vi "GEA2_ICP_Dryer_SM.vi"(0 "ComPort":refnum<visa-resource-name>="COM1", 1 "Destination Address":u8=36 format="%.0x", 2 "Source Address":u8=229 format="%.0x", 5 "Mode":T5=enum."Simulate Dryer", 7 "Xtra Command Data":u8[](array[numeric]) format="%02x", 9 "Dryer Status Serial Data In":T3, 11 "Error In":errorcluster, 13 "Command":T2 items=["CMD_Eval_Mode_Entry_CC1", "CMD_Eval_Mode_Entry_CC2", "CMD_Eval_Mode_Continue", "CMD_Send_DIAG_Info", "CMD_Enable_Debug_Log ", "CMD_Disable_Debug_Log ", "CMD_Send_Log_Data", "CMD_Stop", "RQST_Version"]) -> (4 "Dryer Status Serial Data Out":T3={"Color"=0, "Last Read Status"=enum."Err", "Command:Data"="", "Com Port"=0, "Time(S)"=0.0, "Err Count"=0}, 6 "Read_ACK":bool, 8 "DataReturned":u8[](array[numeric]) format="%.0x", 10 "WriteOK":bool, 14 "CRC Match":bool, 15 "Error Out":errorcluster)   [LabVIEW 2009]
uses:
  GEA2 Dryer Interface Ctrl.ctl
  Dryer Commands.ctl
  Dryer Status Ctrl.ctl
  Dryer Com Port Info.ctl
  <vilib>/Instr/_visa.llb/VISA Configure Serial Port (Instr).vi
  Globals Wilt.vi
  Hybrid Water Heater/HEWH Error Enumeration.ctl
  <vilib>/regexp/Match Regular Expression.xnode
panel:
  out "Remaining States":string
  out "after substring":string
  out "return count 3":u32
  out "Current Read Index":i32
  out "return count":u32
  out "ReadCM2Flag":bool
  out "ReadCM1Flag":bool
  out "Com:Data Buffer":string
  out "Tstart":dbl format="%.2f"
  out "Com:Data":string
  out "CRCArray":u8[](array[numeric]) format="%.0x"
  in  "Tab Control":T1(tab)=enum."Simulate Dryer Data"
  in  "Sim Data":u8[](array[numeric]) format="%02x"
  out "Command Bytes":u8[](array[numeric])=[226, 96, 8, 128, 86, 123, 137, 227] format="%.0x"
  out "ACK(E1?)":u8[](array[numeric]) format="%.0x"
  out "Message Out":u8[](array[numeric]) format="%.0x"
  out "Length":u8
  out "Source Read":u8 format="%.0x"
  out "Destination Read":u8 format="%.0x"
  out "ReadArray":u8[](array[numeric]) format="%.0x"
  out "Bytes At Port":u32=40
  out "CRCRead":u8[](array[numeric]) format="%.0x"
  out "CRC Calc":u8[](array[numeric]) format="%.0x"
  out "Timeout":bool
  out "Num Messages":dbl
  out "Read Pulse":dbl
  out "Time Array":i32[](array[numeric])
  out "Tdiff":i32[](array[numeric])
  out "tStart":u32
  out "State Array":string[](array[string])
  out "Total mS":i32
  in  "Debug":bool
  out "Message for Me":bool
  out "read buffer":string
  out "Partial Message":bool
  out "Send Array":string
  in  "Dryer Status 2 Send":T4
  out "STATUS ACK":bool
  out "ASCII ACK":bool
  out "Status Count":dbl
  out "ASCII Count":dbl
  in  "Period of STATUS (Counts)":dbl=60.0
  in  "Period of Send(mS)":i32=1000
  in  "Enable Read ACK?":bool
  out "Timeout ACK":bool
  in  "Cycle Time (s)":dbl=1000.0 format="%.2f"
  out "Time Left":dbl
  in  "Sim Dryer Start":bool
  out "Drying":bool=TRUE
  out "Sim Init":bool
  out "Start Pressed":bool
  out "Wait Restart":bool
  in  "Serial Timeout":u32=10
  in  "Exit":bool
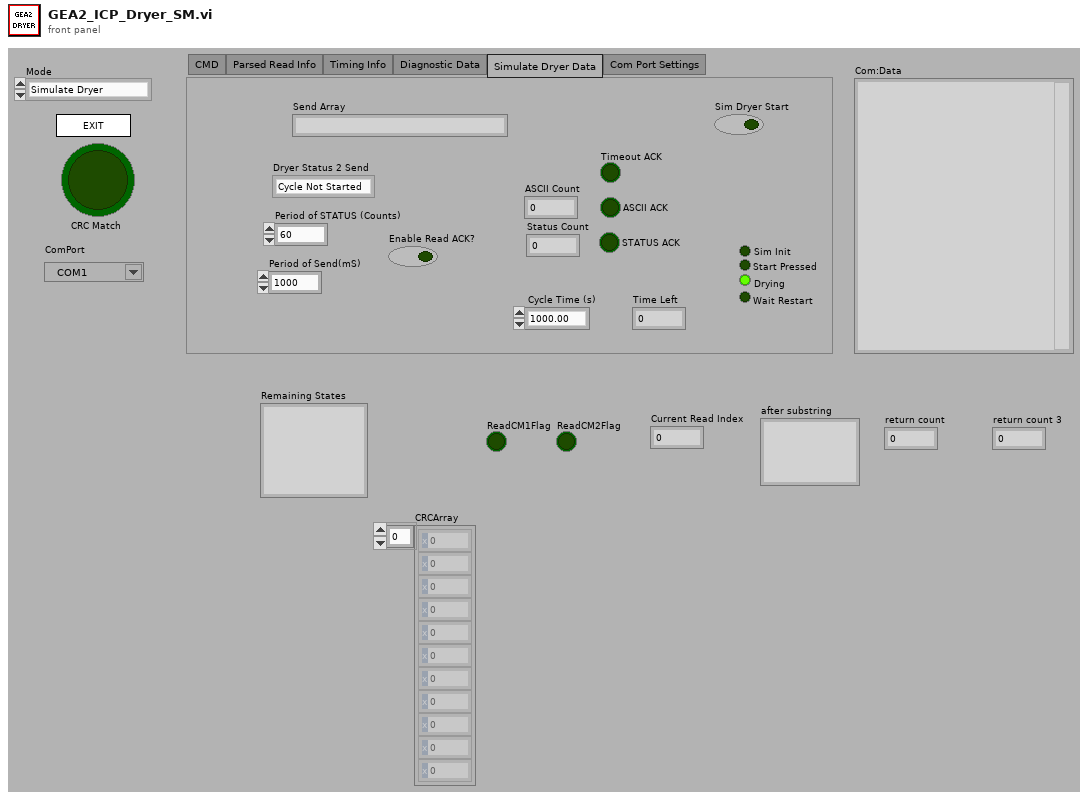
[diagram p1: front panel]
types:
  T1 = enum32{"CMD", "Parsed Read Info", "Timing Info", "Diagnostic Data", "Simulate Dryer Data", "Com Port Settings"}
  T2 = typedef "Dryer Commands.ctl" = u8
  T3 = typedef "Dryer Com Port Info.ctl" = cluster{"Color":u32, "Last Read Status":T4, "Command:Data":string, "Com Port":u8, "Time(S)":dbl, "Err Count":u32}
  T4 = typedef "Dryer Status Ctrl.ctl" = enum16{"Cycle Not Started", "Cycle Running", "Paused", "Cycle Completed", "Eval Mode Entered", "Err"}
  T5 = typedef "GEA2 Dryer Interface Ctrl.ctl" = enum16{"Init Com Port", "SendCMD", "ReadPort", "Close Port", "Simulate Diag Data", "Simulate Dryer", "Send WILT Startup CMDs", "Send Continue CMD", "Read Continuous"}
  T6 = enum32{"invalid app kind", "Development System", "Run Time System", "Student Edition", "Embedded LabVIEW", "Evaluation", "Custom"}
  T7 = enum32{"Invalid", "Standard", "Closed", "Hidden", "Minimized", "Maximized"}
  T8 = typedef "HEWH Error Enumeration.ctl" = enum16{"No Error", "GEA2 Send ACK Mismatch", "GEA2 STX", "GEA2 ETX", "GEA2 CRC Mismatch", "GEA2 ReadACK", "RTD In Range Error", "Fail Mean Tank Temp", "No Flow Config Data Found", "Failed Flow During Purge", "Temp During Purge", "Confirm IF Stop Fail", "Init Draw: TC_1 Out of Range", "Flow = 0 During Draw after 20s"}
  T9 = cluster{"Core":cluster{"Current VI Reference":refnum<vi>, "Close Panel on Exit?":bool}, "ComPort":refnum<visa-resource-name>, "ReadArray":u8[], "CRCArray":u8[], "Bytes Remaining":u8, "CRCRead":u8[], "CRC":bool, "Dryer Command":T2, "Error Out Flag":bool, "Bytes Data":u8[], "Dryer Status Serial Data In":T3, "Current Read Index":i32, "Total Bytes Read":i32, "Reset MSG Count":bool, "ACK":bool, "ReadCM1Flag":bool, "ReadCM2Flag":bool, "Reset Pulse":bool}
  T10 = cluster{"Current VI Reference":refnum<vi>, "Close Panel on Exit?":bool}
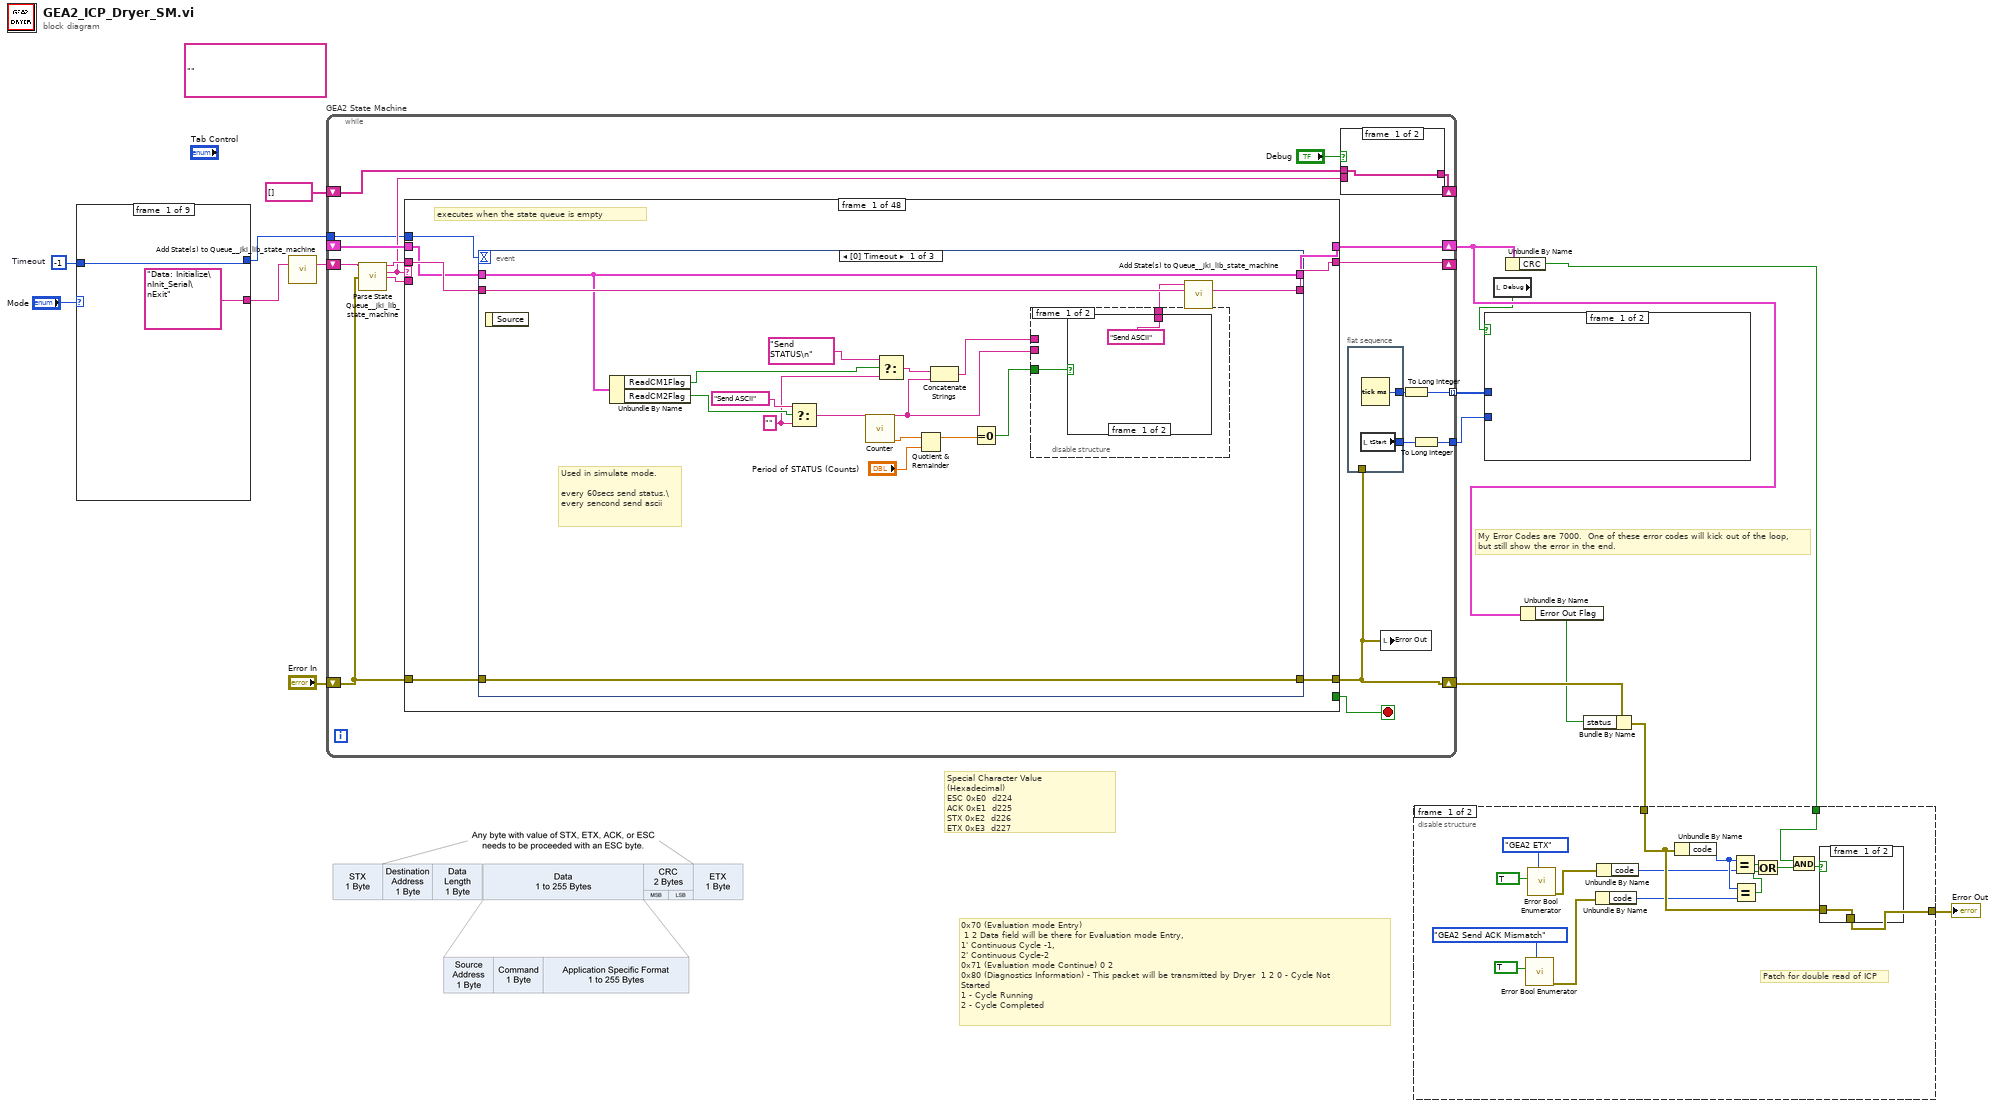
[diagram p0: block diagram]
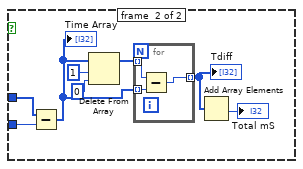
[diagram p2: hidden frame]
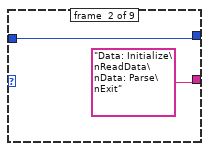
[diagram p3: hidden frame]
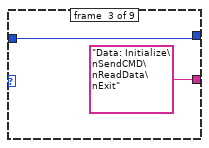
[diagram p4: hidden frame]
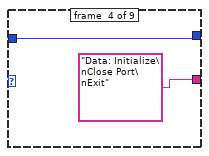
[diagram p5: hidden frame]
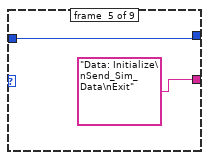
[diagram p6: hidden frame]
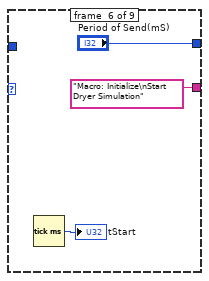
[diagram p7: hidden frame]
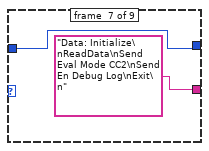
[diagram p8: hidden frame]
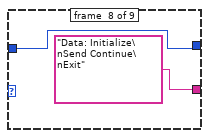
[diagram p9: hidden frame]
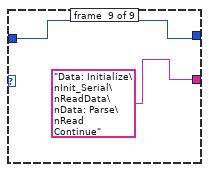
[diagram p10: hidden frame]
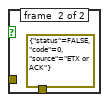
[diagram p11: hidden frame]
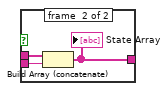
[diagram p13: hidden frame]
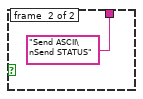
[diagram p14: hidden frame]
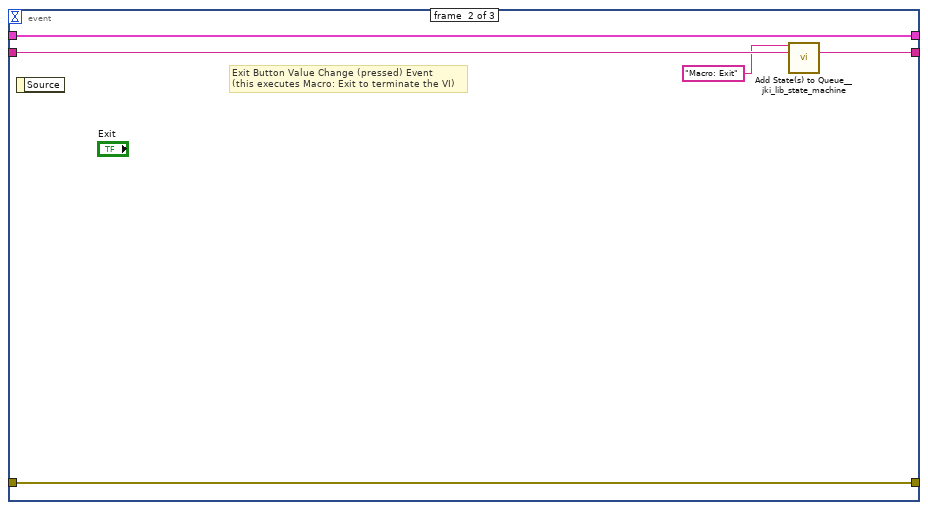
[diagram p17: hidden frame]
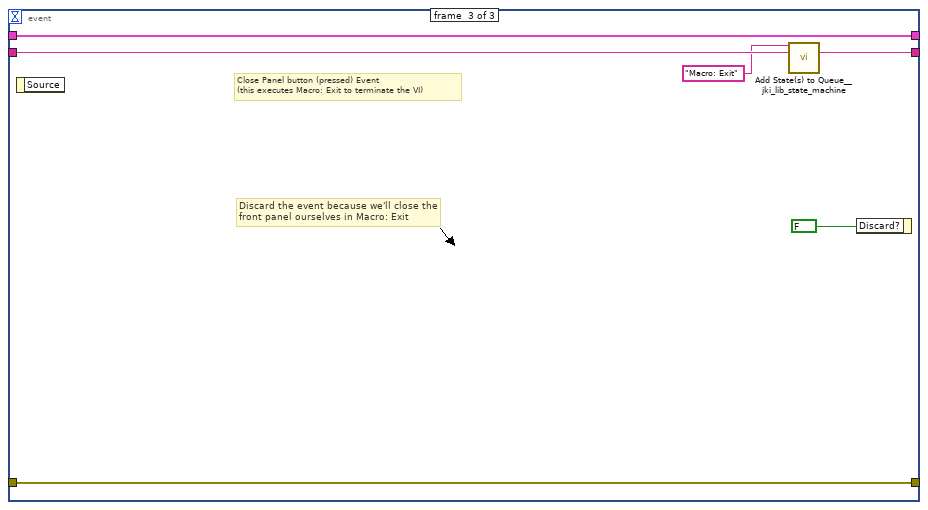
[diagram p18: hidden frame]
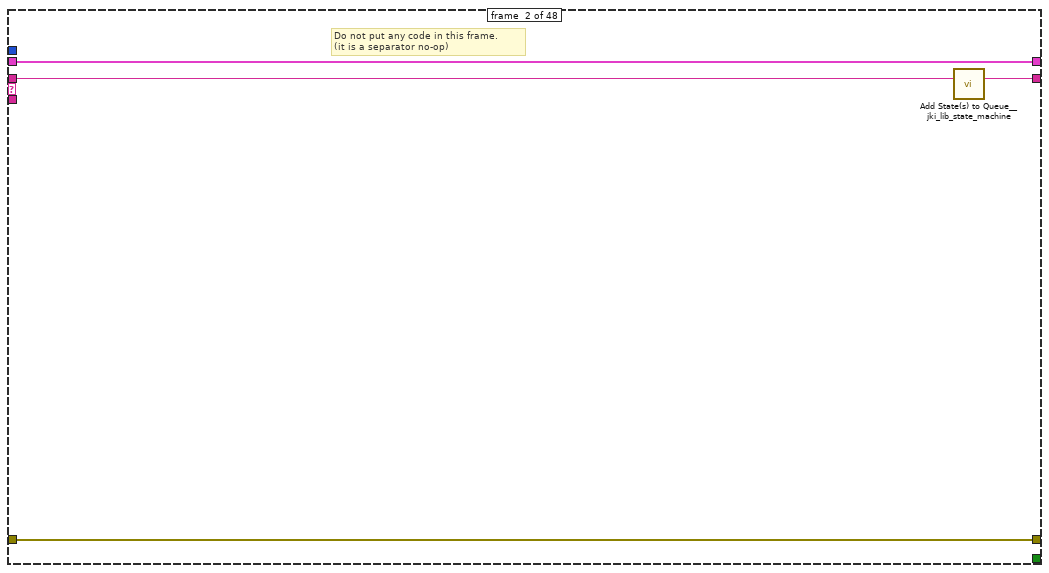
[diagram p19: hidden frame]
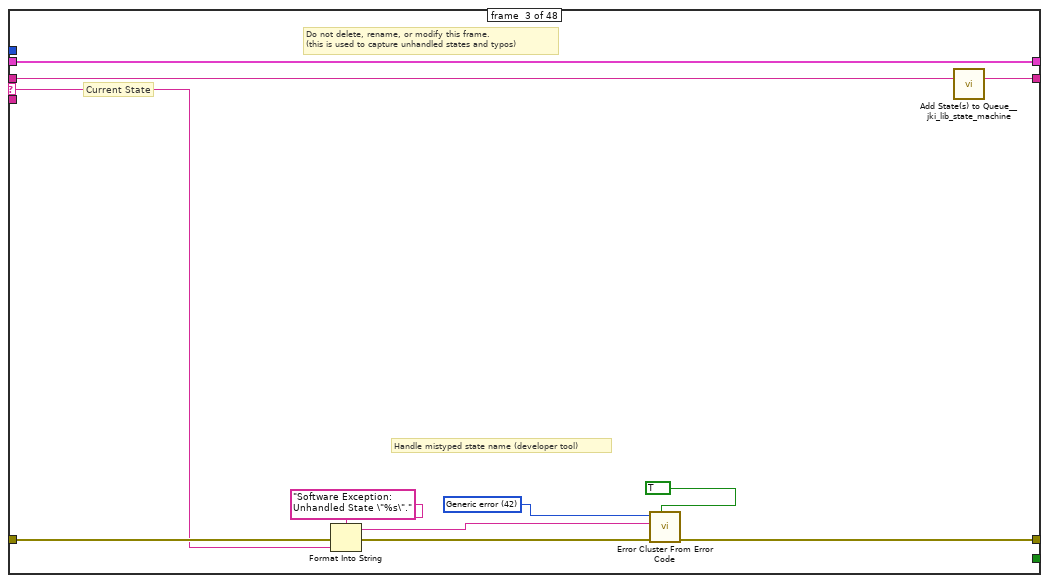
[diagram p20: hidden frame]
diagram:
  (unwired) ""
  w3 = -1  # Timeout
  # "0x70 (Evaluation mode Entry) \n\t1\t2\tData field will be there for Evaluation mode Entry, \n1' Continuous Cycle -1, \n2' Continuous Cycle-2\n0x71 (Evaluation mode Continue)\t0\t2\t\n0x80 (Diagnostics Information) - This packet will be transmitted by Dryer \t1\t2\t0 - Cycle Not Started\n1 - Cycle Running\n2 - Cycle Completed"
  # "My Error Codes are 7000.  One of these error codes will kick out of the loop,\nbut still show the error in the end."
  # "Special Character\tValue (Hexadecimal)\nESC\t0xE0  d224\nACK\t0xE1  d225\nSTX\t0xE2  d226\nETX\t0xE3  d227"
  n1 = case shown="\"ReadPort\", Default" "Mode" {
    tunnel: ["Data: Initialize\nInit_Serial\nExit" "Data: Initialize\nReadData\nData: Parse\nExit" "Data: Initialize\nSendCMD\nReadData\nExit" "Data: Initialize\nClose Port\nExit" "Data: Initialize\nSend_Sim_Data\nExit" "Macro: Initialize\nStart Dryer Simulation" "Data: Initialize\nReadData\nSend Eval Mode CC2\nSend En Debug Log\nExit\n" "Data: Initialize\nSend Continue\nExit" "Data: Initialize\nInit_Serial\nReadData\nData: Parse\nRead Continue"] -> w1
    tunnel: [w17 w19 w21 w23 w25 "Period of Send(mS)" w30 w32 w35] -> w4
    tunnel: w3 -> [w17 w19 w21 w23 w25 _ w30 w32 w35]
    frame #0 {
    }
    frame #1 {
    }
    frame #2 {
    }
    frame #3 {
    }
    frame #4 {
    }
    frame #5 {
      n2 = Tick Count (ms)() -> (millisecond timer value=→"tStart":u32)
    }
    frame #6 {
    }
    frame #7 {
    }
    frame #8 {
    }
  }
  n3 = call <vilib>:"Add State(s) to Queue__jki_lib_state_machine.vi"("State(s) in (\"\")"=w1) -> ("States Out"=w16:string)  [unwired: 14 in]
  n4 = while "GEA2 State Machine" {
    shift-right: [w49] -> w7
    shift-left: _ -> [w48]
    shift-right: [w45] -> w14
    shift-left: "Error In" -> [w47]
    shift-right: [w46] -> _
    shift-left: w16 -> [w51]
    tunnel: [w42] -> w13 mode=indexing
    tunnel: [w41] -> w12
    shift-right: [w38] -> _
    shift-left: string[] [] -> [w40]
    tunnel: w4 -> [w37]
    stop <- w50 stop-if-true
    n5 = call <vilib>:"Parse State Queue__jki_lib_state_machine.vi"("State Queue"=w51, "Error In (no error)"=w47) -> ("Remaining States"=w53:string, "Current State"=w39:string, "Arguments"=w52:string)  [unwired: 11 in]
    n6 = case shown="\"ReadData\"" w39 {
      selector: w39 -> [_ _ w109 _ _ _ _ _ _ _ _ _ _ _ _ _ _ _ _ _ _ _ _ _ _ _ _ _ _ _ _ _ _ _ _ _ _ _ _ _ _ _ _ _ _ _ _ _]
      tunnel: w53 -> [w66 w108 w113 w131 w147 w149 w164 w192 w199 w204 w208 w214 w225 w251 w256 w261 w272 w299 w324 w371 w409 w444 w481 w491 w548 w628 w663 w671 w679 w704 w740 w759 w803 w832 w853 w874 w890 w903 w916 w952 w966 w992 w1004 w1009 w1033 w1267 w1283 w1322]
      tunnel: w52 -> [_ _ _ _ _ _ _ _ _ _ _ w209 w219 _ _ _ _ _ _ _ _ _ _ _ _ _ _ _ _ _ _ _ _ _ _ _ _ _ _ _ _ _ _ _ _ _ _ _]
      tunnel: w48 -> [w64 w105 w111 w122 w143 w152 w161 _ w196 w201 w206 w212 w221 w248 w253 w258 w269 w296 w321 w343 w380 w421 w458 w486 w543 w606 w660 w668 w673 w702 w738 w775 w801 w830 w851 w872 w885 w901 w911 w946 w955 w973 w1001 w1006 w1017 w1262 w1279 w1318]
      tunnel: [w63 w106 w115 w128 w145 w153 w162 w178 w194 w202 w205 w210 w222 w249 w254 w259 w270 w297 w322 w348 w374 w412 w445 w487 w544 w611 w646 w669 w677 w699 w734 w772 w795 w826 w847 w868 w883 w898 w912 w950 w964 w990 w1002 w1007 w1031 w1265 w1282 w1320] -> w45
      tunnel: w47 -> [w62 w106 w114 w128 w139 w153 w162 w178 w197 w202 w205 w211 w223 w249 w254 w259 w270 w282 w317 w350 w393 w427 w464 w488 w545 w613 w643 w669 w677 w696 w734 w772 w795 w826 w847 w868 w888 w895 w914 w950 w964 w990 w1002 w1007 w1031 w1265 w1282 w1320]
      tunnel: [w65 w107 w112 w130 w146 w154 w163 w191 w198 w203 w207 w213 w224 w250 w255 w260 w271 w298 w323 w370 w408 w443 w480 w490 w547 w627 w662 w670 w678 w703 w739 w776 w802 w831 w852 w873 w889 w902 w915 w951 w965 w991 w1003 w1008 w1032 w1266 w1275 w1321] -> w46
      tunnel: [_ _ _ _ _ w150 _ _ _ _ _ _ _ _ _ _ _ _ _ _ _ _ _ _ _ _ _ _ _ _ _ _ _ _ _ _ _ _ _ _ _ _ _ _ _ _ _ _] -> w50
      tunnel: [w61 w105 w111 w129 w142 w152 w161 w190 w196 w201 w206 w212 w221 w248 w253 w258 w269 w295 w320 w343 w379 w421 w458 w486 w543 w606 w653 w668 w672 w701 w737 w774 w800 w829 w850 w871 w884 w900 w911 w945 w954 w989 w1001 w1006 w1014 w1262 w1279 w1318] -> w49
      tunnel: w37 -> [w60 _ _ _ _ _ _ _ _ _ _ _ _ _ _ _ _ _ _ _ _ _ _ _ _ _ _ _ _ _ _ _ _ _ _ _ _ _ _ _ _ _ _ _ _ _ _ _]
      frame #0 {
        # "executes when the state queue is empty"
        n7 = event shown="[0] Timeout" {
          selector: _ -> [_ _ _]
          dyn-events: _ -> [_ _ _]
          timeout: w60 -> [_ _ _]
          tunnel: w66 -> [w83 w98 w104]
          tunnel: [w82 w97 w103] -> w65
          tunnel: w64 -> [w75 w95 w101]
          tunnel: [w81 w96 w102] -> w63
          tunnel: w62 -> [w81 w96 w102]
          tunnel: [w75 w95 w101] -> w61
          event #0 {
            w71 = "" ("f")
            # "Used in simulate mode.\n\nevery 60secs send status.\\\nevery sencond send ascii"
            n8 = event-data() -> ()  [unwired: 1 in, 1 out]
            n9 = Unbundle By Name(w75) -> ("ReadCM1Flag"=w70:bool, "ReadCM2Flag"=w73:bool)
            n10 = Select(t="Send ASCII" ("State(s) in Front (\"\")"), s=w73, f=w71) -> (s? t:f=w68:string)
            n11 = call "Counter.vi"() -> ("Count"=w79:dbl)  [unwired: 11 in]
            n12 = Select(t="Send STATUS\n" ("State(s) in Front (\"\")"), s=w70, f=w71) -> (s? t:f=w69:string)
            n13 = Quotient & Remainder(x=w79, y="Period of STATUS (Counts)") -> (x-y*floor(x/y)=w77:dbl)  [unwired: 1 out]
            n14 = Concatenate Strings(w69, w68) -> (w67:string)
            n15 = Equal To 0?(x=w77) -> (x = 0?=w76:bool)
            n16 = disable-structure shown="Enabled" {
              disable-tunnel: [w85 w90] -> w80
              disable-tunnel: w76 -> [w84 w91]
              disable-tunnel: w68 -> [_ w89]
              disable-tunnel: w67 -> [_ w88]
              frame #0 {
                n17 = case shown="False" w84 {
                  tunnel: ["Send ASCII" ("State(s) in Front (\"\")") "Send ASCII\nSend STATUS" ("State(s) in Front (\"\")")] -> w85
                  frame #0 {
                  }
                  frame #1 {
                  }
                }
              }
              frame #1 {
                n18 = case shown="False" w91 {
                  tunnel: [w92 w93] -> w90
                  tunnel: w89 -> [w92 _]
                  tunnel: w88 -> [_ w93]
                  frame #0 {
                  }
                  frame #1 {
                  }
                }
              }
            }
            n19 = call <vilib>:"Add State(s) to Queue__jki_lib_state_machine.vi"("State(s) in Front (\"\")"=w80, "State(s) in (\"\")"=w83) -> ("States Out"=w82:string)  [unwired: 13 in]
          }
          event #1 {
            # "Exit Button Value Change (pressed) Event\n(this executes Macro: Exit to terminate the VI)"
            n20 = event-data() -> ()  [unwired: 1 in, 1 out]
            n21 = call <vilib>:"Add State(s) to Queue__jki_lib_state_machine.vi"("State(s) in Front (\"\")"="Macro: Exit", "State(s) in (\"\")"=w98) -> ("States Out"=w97:string)  [unwired: 13 in]
          }
          event #2 {
            # "Discard the event because we'll close the front panel ourselves in Macro: Exit"
            # "Close Panel button (pressed) Event\n(this executes Macro: Exit to terminate the VI)"
            n22 = event-data() -> ()  [unwired: 1 in, 1 out]
            n23 = call <vilib>:"Add State(s) to Queue__jki_lib_state_machine.vi"("State(s) in Front (\"\")"="Macro: Exit", "State(s) in (\"\")"=w104) -> ("States Out"=w103:string)  [unwired: 13 in]
            n24 = event-data("Discard?"=FALSE) -> ()  [unwired: 1 in, 1 out]
          }
        }
      }
      frame #1 {
        # "Do not put any code in this frame.\n(it is a separator no-op)"
        n25 = call <vilib>:"Add State(s) to Queue__jki_lib_state_machine.vi"("State(s) in (\"\")"=w108) -> ("States Out"=w107:string)  [unwired: 14 in]
      }
      frame #2 {
        w118 = 42 items=["No error", "Argument error", "Memory is full", "Out of zone", "End of file", "File already open", "Generic file I/O error", "File not found", "File permission error", "Disk is full", "Duplicate path", "Too many files open", "System feature not enabled", "Resource file not found", "Cannot add resource", "Resource not found", "Image not found", "Image memory error", "Pen does not exist", "Config type invalid", "Config token not found", "Config parse error", "Config memory error", "Bad external code format", "Bad external code offset", "External code not present", "Null window", "Destroy window error", "Null menu", "Print aborted", "Bad print record", "Print driver error", "Windows error during printing", "Memory error during printing", "Print dialog error", "Generic print error", "Invalid device refnum", "Device not found", "Device parameter error", "Device unit error", "Cannot open device", "Device call aborted", "Generic error", "Cancelled by user", "Object ID too low", "Object ID too high", "Object not in heap", "Unknown heap", "Unknown object (invalid DefProc)", "Unknown object (DefProc not in table)", "Message out of range", "Invalid (null) method", "Unknown message", "Manager call not supported", "Bad address", "Network operation in progress", "Network operation timed out", "Connection is busy", "Network attribute not supported", "Network error", "Address in use", "System out of memory", "Connection aborted", "Connection refused", "Not connected", "Already connected", "Connection closed", "Initialization error (interapplication manager)", "Bad occurrence", "Wait on unbound occurrence handler", "Occurrence queue overflow", "Datalog type conflict", "Unused", "Unrecognized type (interapplication manager)", "Memory corrupt", "Failed to make temporary DLL", "Old CIN version", "Drag socket not found", "Failed to load drop-object", "Failed to register OLE object", "Failed to release OLE object", "Format specifier type mismatch", "Unknown format specifier", "Too few format specifiers", "Too many format specifiers", "Scan failed", "Newer CIN version", "Error converting to variant", "Runtime menu error", "Password tampered", "Variant attribute not found", "Incompatible variant data type", "Event data is not available", "Event Store is not present", "Occurrence is not found", "Event Queue is not created", "Event info is not available", "Refnum passed is NULL", "Error retrieving Class GUID", "Error retrieving CoClass GUID", "Error retrieving TypeLib GUID.", "Bad built application magic bytes.", "Specific driver is different from the specific driver associated with the Logical Name.", "There is no session opened to the class driver.", "Max Error", "MAX - Error with config objects", "MAX - Error loading configuration", "MAX - Group not supported"]
        # "Current State"
        # "Do not delete, rename, or modify this frame.\n(this is used to capture unhandled states and typos)"
        # "Handle mistyped state name (developer tool)"
        n26 = Format Into String(format string="Software Exception: Unhandled State \"%s\"." ("message"), error in=w114, w109) -> (resulting string=w117:string, error out=w116:errorcluster)  [unwired: 1 in]
        n27 = call <vilib>:"Error Cluster From Error Code.vi"("show call chain? (False)"=TRUE, "error in (no error)"=w116, "error message (\"\")"=w117, "error code (0)"=w118) -> ("error out"=w115:errorcluster)  [unwired: 5 in]
        n28 = call <vilib>:"Add State(s) to Queue__jki_lib_state_machine.vi"("State(s) in (\"\")"=w113) -> ("States Out"=w112:string)  [unwired: 14 in]
      }
      frame #3 {
        # "Do not delete, rename, or modify this frame.\n(this is used to determine panel behavior on exit)"
        # "originally closed?"
        # "exe?"
        # "If panel starts closed or is an EXE, then close it when we exit"
        n29 = property class="VI"() -> ("Front Panel.Open"=w127:bool)  [unwired: 2 in, 2 out]
        n30 = control-ref of="Current VI Reference"() -> (w120:refnum<vi>)
        n31 = property class="App"() -> ("App.Kind"=w126:T6)  [unwired: 2 in, 2 out]
        n32 = Not(x=w127) -> (.not. x?=w124:bool)
        n33 = Equal?(x=w126, y=T6."Run Time System" ("Application:Kind")) -> (x = y?=w123:bool)
        n34 = Or(x=w124, y=w123) -> (x .or. y?=w121:bool)
        n35 = Bundle By Name(cluster=w122, "Core.Current VI Reference"=w120, "Core.Close Panel on Exit?"=w121) -> (w129:T9)
        n36 = call <vilib>:"Add State(s) to Queue__jki_lib_state_machine.vi"("State(s) in (\"\")"=w131) -> ("States Out"=w130:string)  [unwired: 14 in]
      }
      frame #4 {
        # "State Machine Does not handle having an error status = true."
        n37 = local read "ReadArray"() -> (w136:u8[])
        n38 = Unbundle By Name(w139) -> ("source"=w138:string)
        n39 = Number To Hexadecimal String(2:w136) -> (0:w135:string[])  [unwired: 1 in]
        n40 = Array To Spreadsheet String(array=w135, 3:"" ("format string")) -> (spreadsheet string=w133:string)  [unwired: 1 in]
        n41 = Concatenate Strings(w138, ":: BYTES :: " ("string"), w133) -> (w132:string)
        n42 = Bundle By Name(cluster=w143, "Error Out Flag"=TRUE) -> (w142:T9)
        n43 = Bundle By Name(cluster=w139, "source"=w132, "status"=FALSE) -> (w145:errorcluster)
        n44 = call <vilib>:"Add State(s) to Queue__jki_lib_state_machine.vi"("State(s) in Front (\"\")"="Exit", "State(s) in (\"\")"=w147) -> ("States Out"=w146:string)  [unwired: 13 in]
      }
      frame #5 {
        # "Do not put any code in this frame.\n(No errors that occur here will be handled.)"
        n45 = local read "Mode"() -> (w151:T5)
        n46 = case shown="\"Simulate Dryer\"" w151 {
          tunnel: [TRUE w160] -> w150
          tunnel: w149 -> [w155 w159]
          tunnel: [w155 w157] -> w148
          frame #0 {
          }
          frame #1 {
            (unwired) "SendACK" ("regular expression")
            n47 = Match Pattern(string=w159, regular expression="Check Complete") -> (after substring=w157:string)  [unwired: 1 in, 3 out]
            "after substring" <- w157
            n48 = local read "Exit"() -> (w160:bool)
            "Remaining States" <- w159
          }
        }
        n49 = call <vilib>:"Add State(s) to Queue__jki_lib_state_machine.vi"("State(s) in (\"\")"=w148) -> ("States Out"=w154:string)  [unwired: 14 in]
      }
      frame #6 {
        # "Do not put any code in this frame.\n(It is a separator no-op. You can make a copy of this frame to create a new Data frame)"
        n50 = call <vilib>:"Add State(s) to Queue__jki_lib_state_machine.vi"("State(s) in (\"\")"=w164) -> ("States Out"=w163:string)  [unwired: 14 in]
      }
      frame #7 {
        w165 = FALSE ("Start Pressed")
        w166 = TRUE  # Reset Pulse
        w169 = FALSE  # ReadCM2Flag
        w170 = FALSE  # ReadCM1Flag
        w167 = "" ("Com:Data")
        w171 = FALSE  # ACK
        w172 = TRUE  # Reset MSG Count
        w173 = 0  # Total Bytes Read
        w174 = 0  # Current Read Index
        w179 = u8 0 ("Length")
        w180 = T2 3 items=["Eval_Mode_Entry_CC1", "Eval_Mode_Entry_CC2", "Eval_Mode_Continue", "Get_Diagnostic_Info"]  # Dryer Command
        w181 = u8[] []  # Bytes Data
        w182 = T10 {"Current VI Reference"=refnum, "Close Panel on Exit?"=FALSE}  # Core
        w168 = FALSE ("CRC Match")
        w183 = FALSE  # Error Out Flag
        w184 = FALSE  # CRC
        w185 = u8[] []  # CRCRead
        w186 = u8 0  # Bytes Remaining
        w187 = u8[] []  # CRCArray
        w188 = u8[] []  # ReadArray
        # "Don' Run with Err In"
        # "Initialize the shift-register data, here.\n(data names are defined by what you wire into the bundle function)"
        n51 = local write "Com:Data Buffer"(w167) -> ()
        n52 = local write "Num Messages"(0.0 ("Num Messages")) -> ()
        n53 = local write "Com:Data"(w167) -> ()
        n54 = local write "Wait Restart"(w165) -> ()
        n55 = local write "Sim Init"(w165) -> ()
        n56 = local write "Start Pressed"(w165) -> ()
        n57 = local write "Drying"(w165) -> ()
        n58 = local write "ReadCM2Flag"(w165) -> ()
        n59 = local write "Exit"(w165) -> ()
        n60 = local write "ReadCM1Flag"(w165) -> ()
        n61 = local write "Source Read"(w179) -> ()
        n62 = local write "Length"(w179) -> ()
        n63 = local write "Message for Me"(w168) -> ()
        n64 = local write "Message for Me"(w168) -> ()
        n65 = local write "CRC Match"(w168) -> ()
        n66 = local write "WriteOK"(w168) -> ()
        n67 = local write "Read_ACK"(w168) -> ()
        n68 = local write "Timeout"(w168) -> ()
        n69 = local write "Partial Message"(w168) -> ()
        n70 = local write "Drying"(w168) -> ()
        n71 = Bundle("Core"=w182, "ComPort"="ComPort", "ReadArray"=w188, "CRCArray"=w187, "Bytes Remaining"=w186, "CRCRead"=w185, "CRC"=w184, "Dryer Command"=w180, "Error Out Flag"=w183, "Bytes Data"=w181, "Dryer Status Serial Data In"="Dryer Status Serial Data In", "Current Read Index"=w174, "Total Bytes Read"=w173, "Reset MSG Count"=w172, "ACK"=w171, "ReadCM1Flag"=w170, "ReadCM2Flag"=w169, "Reset Pulse"=w166) -> (w190:T9)  [unwired: 1 in]
        n72 = case shown="Error" w178 {
          tunnel: [_ "Exit"] -> w177
          frame #0 {
          }
          frame #1 {
          }
        }
        n73 = call <vilib>:"Add State(s) to Queue__jki_lib_state_machine.vi"("State(s) in Front (\"\")"=w177, "State(s) in (\"\")"=w192) -> ("States Out"=w191:string)  [unwired: 13 in]
        "Com:Data Buffer" <- w167
      }
      frame #8 {
        # "Cleanup any data and references, here.\n(this is called automatically, by the Macro: Exit)"
        n74 = Unbundle By Name(w196) -> ("Core.Current VI Reference"=w195:refnum<vi>)
        n75 = Close Reference(reference=w195, error in (no error)=w197) -> (error out=w194:errorcluster)
        n76 = case shown="Error" w194 {
          frame #0 {
          }
          frame #1 {
            n77 = String Length(string="") -> ()  [unwired: 1 out]
          }
        }
        n78 = call <vilib>:"Add State(s) to Queue__jki_lib_state_machine.vi"("State(s) in (\"\")"=w199) -> ("States Out"=w198:string)  [unwired: 14 in]
      }
      frame #9 {
        # "Do not put any code in this frame.\n(It is a separator no-op. You can make a copy of this frame to create a new UI frame)"
        n79 = call <vilib>:"Add State(s) to Queue__jki_lib_state_machine.vi"("State(s) in (\"\")"=w204) -> ("States Out"=w203:string)  [unwired: 14 in]
      }
      frame #10 {
        # "Initialize the User Interface, here.\n(this is called automatically, by the Macro: Init)"
        n80 = call <vilib>:"Add State(s) to Queue__jki_lib_state_machine.vi"("State(s) in (\"\")"=w208) -> ("States Out"=w207:string)  [unwired: 14 in]
      }
      frame #11 {
        # "Argument"
        # "Set and Unset Cursor Busy.\n(Usage: \"UI: Cursor Set >> Busy|Idle\")"
        n81 = case shown="\"Idle\", Default" w209 {
          tunnel: w211 -> [w216 w218]
          tunnel: [w215 w217] -> w210
          frame #0 {
            n82 = call <vilib>:"Unset Busy.vi"("error in (no error)"=w216) -> ("error out"=w215:errorcluster)  [unwired: 10 in]
          }
          frame #1 {
            n83 = call <vilib>:"Set Busy.vi"("error in (no error)"=w218) -> ("error out"=w217:errorcluster)  [unwired: 9 in, 1 out]
          }
        }
        n84 = call <vilib>:"Add State(s) to Queue__jki_lib_state_machine.vi"("State(s) in (\"\")"=w214) -> ("States Out"=w213:string)  [unwired: 14 in]
      }
      frame #12 {
        # "Argument"
        # "Set Front Panel Open or Closed\n(Usage: \"UI: Front Panel State >> Open|Close\")"
        n85 = Unbundle By Name(w221) -> ("Core.Current VI Reference"=w220:refnum<vi>)
        n86 = case shown="\"Close\"" w219 {
          tunnel: w223 -> [w229 w242]
          tunnel: [w231 w243] -> w222
          tunnel: w220 -> [w230 w240]
          frame #0 {
            n87 = property class="VI"(reference=w230, error in=w229) -> (reference out=w227:refnum<vi>, error out=w228:errorcluster, "Front Panel.Open"=w226:bool)
            n88 = case shown="False" w226 {
              tunnel: [w234 w237] -> w231
              tunnel: w228 -> [w233 w237]
              tunnel: w227 -> [w232 _]
              frame #0 {
                n89 = invoke class="VI" method="FP.Open"(reference=w232, error in=w233, "Activate"=TRUE, "State"=T7."Standard") -> (error out=w234:errorcluster)  [unwired: 1 in, 4 out]
              }
              frame #1 {
              }
            }
          }
          frame #1 {
            n90 = property class="VI"(reference=w240, error in=w242) -> (reference out=w239:refnum<vi>, error out=w241:errorcluster, "Front Panel.Open"=w238:bool)
            n91 = case shown="True" w238 {
              tunnel: [w244 w247] -> w243
              tunnel: w241 -> [w244 w246]
              tunnel: w239 -> [_ w245]
              frame #0 {
              }
              frame #1 {
                n92 = invoke class="VI" method="FP.Close"(reference=w245, error in=w246) -> (error out=w247:errorcluster)  [unwired: 1 in, 2 out]
              }
            }
          }
        }
        n93 = call <vilib>:"Add State(s) to Queue__jki_lib_state_machine.vi"("State(s) in (\"\")"=w225) -> ("States Out"=w224:string)  [unwired: 14 in]
      }
      frame #13 {
        # "Do not put any code in this frame.\n(It is a separator no-op. You can make a copy of this frame to create a new Macro frame)"
        n94 = call <vilib>:"Add State(s) to Queue__jki_lib_state_machine.vi"("State(s) in (\"\")"=w251) -> ("States Out"=w250:string)  [unwired: 14 in]
      }
      frame #14 {
        w252 = "Data: Initialize\nInitialize Core Data\nUI: Initialize\nUI: Front Panel State >> Open\nInit_Serial"  # Data: Initialize Initialize Core Data UI: Initialize UI: Front Panel State >> Open Init_Serial
        # "Initialization Macro\n(This is called once, when the VI starts)"
        n95 = call <vilib>:"Add State(s) to Queue__jki_lib_state_machine.vi"("State(s) in Front (\"\")"=w252, "State(s) in (\"\")"=w256) -> ("States Out"=w255:string)  [unwired: 13 in]
      }
      frame #15 {
        # "Exit Macro\n(This is called once, when the VI exits)"
        n96 = disable-structure shown="Enabled" {
          disable-tunnel: w258 -> [w268 _]
          disable-tunnel: [w263 _] -> w257
          frame #0 {
            n97 = Unbundle By Name(w268) -> ()  [unwired: 1 out]
            n98 = Select(t="UI: Front Panel State >> Close", s=FALSE, f="") -> (s? t:f=w265:string)
            n99 = call <vilib>:"Add State(s) to Queue__jki_lib_state_machine.vi"("State(s) in (\"\")"=w265, "State(s) at Back (\"\")"="Data: Cleanup\nExit") -> ("States Out"=w263:string)  [unwired: 13 in]
          }
          frame #1 {
          }
        }
        n100 = call <vilib>:"Add State(s) to Queue__jki_lib_state_machine.vi"("State(s) in Front (\"\")"=w257, "State(s) in (\"\")"=w261) -> ("States Out"=w260:string)  [unwired: 13 in]
      }
      frame #16 {
        # "Template Separator\n(You can make a copy of, or modify, this frame)"
        n101 = call <vilib>:"Add State(s) to Queue__jki_lib_state_machine.vi"("State(s) in (\"\")"=w272) -> ("States Out"=w271:string)  [unwired: 14 in]
      }
      frame #17 {
        w289 = u16 0 items=["None", "XON/XOFF", "RTS/CTS", "XON/XOFF & RTS/CTS", "DTR/DSR", "XON/XOFF & DTR/DSR"] ("flow control (0:none)")
        w288 = u16 10 items=["1.0"=10, "1.5"=15, "2.0"=20] ("stop bits (10: 1 bit)")
        # "skip error handle routine"
        # "Assumes that if the serial port is 19200, then it is all ok."
        # "Your code here.\n(You can make a copy of, or modify, this frame)"
        n102 = Unbundle By Name(w296) -> ("ComPort"=w276:refnum<visa-resource-name>)
        n103 = call "Com Chan Type Conversion.vi"("Com Chan In"=w276) -> ("Com Channel #"=w275:u8)  [unwired: 11 in, 3 out]
        n104 = global read "Globals Wilt.vi" "No Com Color"() -> (w281:u32)
        n105 = Bundle By Name(cluster=T3 {"Color"=0, "Last Read Status"=enum."Err", "Command:Data"="", "Com Port"=0, "Time(S)"=0.0, "Err Count"=0} ("Dryer Status Serial Data Out"), "Color"=w281, "Last Read Status"=Dryer_Status_Ctrl."Err", "Command:Data"="", "Com Port"=w275, "Time(S)"=0.0, "Err Count"=u32 0) -> (w274:T3)
        n106 = call-poly "VISA Configure Serial Port"("VISA resource name"=w276, "timeout (10sec)"="Serial Timeout", "Enable Termination\nChar (T)"=FALSE ("Enable Termination\nChar (T)"), "baud rate (9600)"=u32 19200, "data bits (8)"=u16 8, "parity (0:none)"=enum16{"None", "Odd", "Even", "Mark", "Space"}."None", "error in (no error)"=w282, "stop bits (10: 1 bit)"=w288, "flow control (0:none)"=w289) -> ("VISA resource name out"=w292:refnum<visa-resource-name>, "error out"=w293:errorcluster)  [unwired: 5 in]
        n107 = Equal To 0?(x="Serial Timeout") -> (x = 0?=w284:bool)
        n108 = case shown="True" w284 {
          tunnel: w293 -> [w300 w303]
          tunnel: w292 -> [_ w302]
          tunnel: [w300 w301] -> w291
          frame #0 {
          }
          frame #1 {
            n109 = VISA Flush I/O Buffer(VISA resource name=w302, error in (no error)=w303) -> (error out=w301:errorcluster)  [unwired: 1 in, 1 out]
          }
        }
        n110 = local write "Dryer Status Serial Data Out"(w274) -> ()
        n111 = case shown="Error" w291 {
          selector: w291 -> [w304 w311]
          tunnel: w296 -> [w308 w315]
          tunnel: [w307 w314] -> w295
          tunnel: w292 -> [w306 _]
          tunnel: ["" ("State(s) in Front (\"\")") "Exit" ("State(s) in Front (\"\")")] -> w294
          tunnel: [w304 w309] -> w297
          frame #0 {
            n112 = Bundle By Name(cluster=w308, "ComPort"=w306) -> (w307:T9)
          }
          frame #1 {
            n113 = Bundle By Name(cluster=w315, "Error Out Flag"=TRUE) -> (w314:T9)
            n114 = Bundle By Name(cluster=w311, "status"=FALSE) -> (w309:errorcluster)
          }
        }
        n115 = call <vilib>:"Add State(s) to Queue__jki_lib_state_machine.vi"("State(s) in Front (\"\")"=w294, "State(s) in (\"\")"=w299) -> ("States Out"=w298:string)  [unwired: 13 in]
      }
      frame #18 {
        # "skip error handle routine"
        # "Assumes that if the serial port is 19200, then it is all ok."
        # "Your code here.\n(You can make a copy of, or modify, this frame)"
        n116 = Unbundle By Name(w321) -> ("ComPort"=w316:refnum<visa-resource-name>)
        n117 = VISA Close(VISA resource name=w316, error in (no error)=w317) -> (error out=w318:errorcluster)
        n118 = case shown="Error" w318 {
          selector: w318 -> [w326 w330]
          tunnel: w321 -> [w325 w334]
          tunnel: [w325 w333] -> w320
          tunnel: ["" ("State(s) in Front (\"\")") "Macro: Exit" ("State(s) in Front (\"\")")] -> w319
          tunnel: [w326 w328] -> w322
          frame #0 {
          }
          frame #1 {
            n119 = Bundle By Name(cluster=w334, "Error Out Flag"=TRUE) -> (w333:T9)
            n120 = Bundle By Name(cluster=w330, "status"=FALSE) -> (w328:errorcluster)
          }
        }
        n121 = call <vilib>:"Add State(s) to Queue__jki_lib_state_machine.vi"("State(s) in Front (\"\")"=w319, "State(s) in (\"\")"=w324) -> ("States Out"=w323:string)  [unwired: 13 in]
      }
      frame #19 {
        w345 = u8 225  # ACK
        w356 = u8 227  # ETX
        w359 = u8 226  # STX
        n122 = Unbundle By Name(w343) -> ("ComPort"=w369:refnum<visa-resource-name>)
        n123 = call "Dryer_DSM_CMD.vi"("Command"="Command") -> ("CMD Array"=w361:u8[])  [unwired: 10 in]
        n124 = Array Size(array=w361) -> (size(s)=w367:i32)
        n125 = Array Size(array="Xtra Command Data") -> (size(s)=w365:i32)
        n126 = Compound Arithmetic op=ADD(7 ("x"), w367, w365) -> (w363:i32)
        n127 = To Unsigned Byte Integer(number=w363) -> (unsigned 8bit integer=w364:u8)
        n128 = Build Array (concatenate)("Destination Address", w364, "Source Address", w361, "Xtra Command Data") -> (w358:u8[])
        n129 = call "crc16-ccitt (x1021).vi"("unsigned byte array"=w358) -> ("CRC"=w357:u8[])  [unwired: 9 in, 1 out]
        n130 = call "HEWH Command Needs Read.vi"("Command"="Command") -> ("RQST"=w341:bool)  [unwired: 13 in, 1 out]
        n131 = Build Array (concatenate)(w359, w358, w357, w356) -> (w338:u8[])
        n132 = call "GEA2 Add ESC Char.vi"("Message"=w338) -> ("Message Out"=w337:u8[])  [unwired: 14 in]
        "Command Bytes" <- w337
        n133 = Byte Array To String(unsigned byte array=w337) -> (string=w339:string)
        n134 = Array Size(array=w337) -> (size(s)=w352:i32)
        n135 = Increment(x=w352) -> (x+1=w346:i32)
        n136 = VISA Write(VISA resource name=w369, write buffer=w339, error in (no error)=w350) -> (VISA resource name out=w355:refnum<visa-resource-name>, error out=w354:errorcluster)  [unwired: 1 out]
        n137 = To Unsigned Long Integer(number=w346) -> (unsigned 32bit integer=w336:u32)
        n138 = Build Array (concatenate)(w337, w345) -> (w344:u8[])
        n139 = Byte Array To String(unsigned byte array=w344) -> (string=w351:string)
        n140 = VISA Read(VISA resource name=w355, byte count=w336, error in (no error)=w354) -> (read buffer=w335:string, error out=w349:errorcluster)  [unwired: 2 out]
        n141 = Equal?(x=w351, y=w335) -> (x = y?=→"WriteOK":bool)
        n142 = case shown="True" w341 {
          tunnel: ["" "ReadData\nData: Parse\n"] -> w340
          frame #0 {
          }
          frame #1 {
          }
        }
        n143 = call "Delay mS.vi"("Error In"=w349, "milliseconds to wait"=u32 10) -> ("Error Out"=w348:errorcluster)  [unwired: 13 in]
        n144 = call <vilib>:"Add State(s) to Queue__jki_lib_state_machine.vi"("State(s) in Front (\"\")"=w340, "State(s) in (\"\")"=w371) -> ("States Out"=w370:string)  [unwired: 13 in]
      }
      frame #20 {
        w389 = T2 1 items=["CMD_Eval_Mode_Entry_CC1", "CMD_Eval_Mode_Entry_CC2", "CMD_Eval_Mode_Continue", "CMD_Send_DIAG_Info", "CMD_Enable_Debug_Log ", "CMD_Disable_Debug_Log ", "CMD_Send_Log_Data"] ("Command 2")
        w391 = u8 225  # ACK
        w398 = u8 227  # ETX
        w401 = u8 226  # STX
        n145 = Unbundle By Name(w380) -> ("ComPort"=w407:refnum<visa-resource-name>)
        n146 = call "Dryer_DSM_CMD.vi"("Command"=w389) -> ("CMD Array"=w402:u8[])  [unwired: 10 in]
        n147 = local read "Destination Address"() -> (w388:u8)
        n148 = local read "Source Address"() -> (w387:u8)
        n149 = Array Size(array=w402) -> (size(s)=w406:i32)
        n150 = Compound Arithmetic op=ADD(7 ("x"), w406) -> (w403:i32)
        n151 = To Unsigned Byte Integer(number=w403) -> (unsigned 8bit integer=w404:u8)
        n152 = Build Array (concatenate)(w388, w404, w387, w402) -> (w400:u8[])
        n153 = call "crc16-ccitt (x1021).vi"("unsigned byte array"=w400) -> ("CRC"=w399:u8[])  [unwired: 9 in, 1 out]
        n154 = Build Array (concatenate)(w401, w400, w399, w398) -> (w384:u8[])
        n155 = call "GEA2 Add ESC Char.vi"("Message"=w384) -> ("Message Out"=w383:u8[])  [unwired: 14 in]
        "Message Out" <- w383
        n156 = Array Size(array=w383) -> (size(s)=w395:i32)
        n157 = Byte Array To String(unsigned byte array=w383) -> (string=w386:string)
        n158 = VISA Write(VISA resource name=w407, write buffer=w386, error in (no error)=w393) -> (VISA resource name out=w397:refnum<visa-resource-name>, error out=w396:errorcluster)  [unwired: 1 out]
        n159 = Increment(x=w395) -> (x+1=w392:i32)
        n160 = call "Delay mS.vi"("Error In"=w396, "milliseconds to wait"=u32 1000) -> ("Error Out"=w376:errorcluster)  [unwired: 13 in]
        n161 = To Unsigned Long Integer(number=w392) -> (unsigned 32bit integer=w385:u32)
        n162 = Build Array (concatenate)(w383, w391) -> (w390:u8[])
        n163 = Byte Array To String(unsigned byte array=w390) -> (string=w394:string)
        n164 = VISA Read(VISA resource name=w397, byte count=w385, error in (no error)=w376) -> (read buffer=w381:string, return count=→"return count 3":u32, error out=w382:errorcluster)  [unwired: 1 out]
        n165 = Equal?(x=w394, y=w381) -> (x = y?=w378:bool)
        n166 = Bundle By Name(cluster=w380, "ACK"=w378) -> (w379:T9)
        n167 = disable-structure shown="Enabled" {
          disable-tunnel: w382 -> [w411 _]
          disable-tunnel: [w410 _] -> w374
          frame #0 {
            n168 = call <vilib>:"Clear Errors.vi"("error in (no error)"=w411) -> ("error out"=w410:errorcluster)  [unwired: 6 in]
          }
          frame #1 {
          }
        }
        n169 = call <vilib>:"Add State(s) to Queue__jki_lib_state_machine.vi"("State(s) in (\"\")"=w409) -> ("States Out"=w408:string)  [unwired: 14 in]
      }
      frame #21 {
        w420 = T2 2 items=["CMD_Eval_Mode_Entry_CC1", "CMD_Eval_Mode_Entry_CC2", "CMD_Eval_Mode_Continue", "CMD_Send_DIAG_Info", "CMD_Enable_Debug_Log ", "CMD_Disable_Debug_Log ", "CMD_Send_Log_Data"] ("Command 2")
        w423 = u8 225  # ACK
        w433 = u8 227  # ETX
        w436 = u8 226  # STX
        n170 = Unbundle By Name(w421) -> ("ComPort"=w442:refnum<visa-resource-name>)
        n171 = call "Dryer_DSM_CMD.vi"("Command"=w420) -> ("CMD Array"=w437:u8[])  [unwired: 10 in]
        n172 = local read "Source Address"() -> (w418:u8)
        n173 = Array Size(array=w437) -> (size(s)=w441:i32)
        n174 = local read "Destination Address"() -> (w419:u8)
        n175 = Compound Arithmetic op=ADD(7 ("x"), w441) -> (w438:i32)
        n176 = To Unsigned Byte Integer(number=w438) -> (unsigned 8bit integer=w439:u8)
        n177 = Build Array (concatenate)(w419, w439, w418, w437) -> (w435:u8[])
        n178 = call "crc16-ccitt (x1021).vi"("unsigned byte array"=w435) -> ("CRC"=w434:u8[])  [unwired: 9 in, 1 out]
        n179 = Build Array (concatenate)(w436, w435, w434, w433) -> (w416:u8[])
        n180 = call "GEA2 Add ESC Char.vi"("Message"=w416) -> ("Message Out"=w414:u8[])  [unwired: 14 in]
        n181 = Array Size(array=w414) -> (size(s)=w429:i32)
        n182 = Byte Array To String(unsigned byte array=w414) -> (string=w415:string)
        n183 = Increment(x=w429) -> (x+1=w424:i32)
        n184 = VISA Write(VISA resource name=w442, write buffer=w415, error in (no error)=w427) -> (VISA resource name out=w432:refnum<visa-resource-name>, error out=w430:errorcluster)  [unwired: 1 out]
        n185 = To Unsigned Long Integer(number=w424) -> (unsigned 32bit integer=w413:u32)
        n186 = Build Array (concatenate)(w414, w423) -> (w422:u8[])
        n187 = Byte Array To String(unsigned byte array=w422) -> (string=w428:string)
        n188 = VISA Read(VISA resource name=w432, byte count=w413, error in (no error)=w430) -> (read buffer=w431:string, error out=w426:errorcluster)  [unwired: 2 out]
        n189 = Equal?(x=w428, y=w431) -> (x = y?=w417:bool)
        n190 = call "Delay mS.vi"("Error In"=w426, "milliseconds to wait"=u32 100) -> ("Error Out"=w412:errorcluster)  [unwired: 13 in]
        n191 = local write "WriteOK"(w417) -> ()
        n192 = call <vilib>:"Add State(s) to Queue__jki_lib_state_machine.vi"("State(s) in (\"\")"=w444) -> ("States Out"=w443:string)  [unwired: 14 in]
      }
      frame #22 {
        w457 = T2 4 items=["CMD_Eval_Mode_Entry_CC1", "CMD_Eval_Mode_Entry_CC2", "CMD_Eval_Mode_Continue", "CMD_Send_DIAG_Info", "CMD_Enable_Debug_Log ", "CMD_Disable_Debug_Log ", "CMD_Send_Log_Data"] ("Command 2")
        w460 = u8 225  # ACK
        w470 = u8 227  # ETX
        w473 = u8 226  # STX
        n193 = Unbundle By Name(w458) -> ("ComPort"=w479:refnum<visa-resource-name>, "ACK"=w448:bool)
        n194 = call "Dryer_DSM_CMD.vi"("Command"=w457) -> ("CMD Array"=w474:u8[])  [unwired: 10 in]
        n195 = Array Size(array=w474) -> (size(s)=w478:i32)
        n196 = local read "Destination Address"() -> (w456:u8)
        n197 = local read "Source Address"() -> (w455:u8)
        n198 = Compound Arithmetic op=ADD(7 ("x"), w478) -> (w475:i32)
        n199 = To Unsigned Byte Integer(number=w475) -> (unsigned 8bit integer=w476:u8)
        n200 = Build Array (concatenate)(w456, w476, w455, w474) -> (w472:u8[])
        n201 = call "crc16-ccitt (x1021).vi"("unsigned byte array"=w472) -> ("CRC"=w471:u8[])  [unwired: 9 in, 1 out]
        n202 = Build Array (concatenate)(w473, w472, w471, w470) -> (w452:u8[])
        n203 = call "GEA2 Add ESC Char.vi"("Message"=w452) -> ("Message Out"=w451:u8[])  [unwired: 14 in]
        n204 = Build Array (concatenate)(w451, w460) -> (w459:u8[])
        n205 = Array Size(array=w451) -> (size(s)=w466:i32)
        n206 = Increment(x=w466) -> (x+1=w461:i32)
        n207 = Byte Array To String(unsigned byte array=w459) -> (string=w465:string)
        n208 = Byte Array To String(unsigned byte array=w451) -> (string=w454:string)
        n209 = To Unsigned Long Integer(number=w461) -> (unsigned 32bit integer=w453:u32)
        n210 = VISA Write(VISA resource name=w479, write buffer=w454, error in (no error)=w464) -> (VISA resource name out=w469:refnum<visa-resource-name>, error out=w467:errorcluster)  [unwired: 1 out]
        n211 = VISA Read(VISA resource name=w469, byte count=w453, error in (no error)=w467) -> (read buffer=w468:string, return count=→"return count":u32, error out=w463:errorcluster)  [unwired: 1 out]
        n212 = Equal?(x=w465, y=w468) -> (x = y?=w450:bool)
        n213 = call "Delay mS.vi"("Error In"=w463, "milliseconds to wait"=u32 500) -> ("Error Out"=w446:errorcluster)  [unwired: 13 in]
        n214 = And(x=w448, y=w450) -> (x .and. y?=w449:bool)
        n215 = disable-structure shown="Enabled" {
          disable-tunnel: w446 -> [w483 _]
          disable-tunnel: [w482 _] -> w445
          frame #0 {
            n216 = call <vilib>:"Clear Errors.vi"("error in (no error)"=w483) -> ("error out"=w482:errorcluster)  [unwired: 6 in]
          }
          frame #1 {
          }
        }
        n217 = local write "WriteOK"(w449) -> ()
        n218 = call <vilib>:"Add State(s) to Queue__jki_lib_state_machine.vi"("State(s) in (\"\")"=w481) -> ("States Out"=w480:string)  [unwired: 14 in]
      }
      frame #23 {
        n219 = call "Counter.vi"() -> ("Count"=w484:dbl)  [unwired: 11 in]
        n220 = Unbundle By Name(w486) -> ("ComPort"=w489:refnum<visa-resource-name>)
        n221 = for {
          N: 2 -> [_]
          tunnel: w489 -> [w531]
          tunnel: w488 -> [w515]
          tunnel: [w514] -> w487
          tunnel: w484 -> [w502]
          stop <- w503 stop-if-true
          w501 = errorcluster {"status"=TRUE, "code"=-1073807339, "source"="VISA Read in GEA2_ICP_Dryer_SM.vi"}  # timeout error
          w510 = T2 6 items=["CMD_Eval_Mode_Entry_CC1", "CMD_Eval_Mode_Entry_CC2", "CMD_Eval_Mode_Continue", "CMD_Send_DIAG_Info", "CMD_Enable_Debug_Log ", "CMD_Disable_Debug_Log ", "CMD_Send_Log_Data"] ("Command")
          w512 = u8 225  # ACK
          w521 = u8 227  # ETX
          w524 = u8 226  # STX
          n222 = call "Dryer_DSM_CMD.vi"("Command"=w510) -> ("CMD Array"=w525:u8[])  [unwired: 10 in]
          n223 = local read "Destination Address"() -> (w504:u8)
          n224 = Array Size(array=w525) -> (size(s)=w530:i32)
          n225 = local read "Source Address"() -> (w505:u8)
          n226 = Quotient & Remainder(x=w502, y=32.0) -> (x-y*floor(x/y)=w506:dbl)  [unwired: 1 out]
          n227 = String To Byte Array(string="1234567890ABCDEFGHIJKLMNOPQRSTUV") -> (unsigned byte array=w508:u8[])
          n228 = Rotate 1D Array(1:w508, 2:w506) -> (0:w497:u8[])
          n229 = Array Size(array=w497) -> (size(s)=w528:i32)
          n230 = Compound Arithmetic op=ADD(7 ("x"), w530, w528) -> (w526:i32)
          n231 = To Unsigned Byte Integer(number=w526) -> (unsigned 8bit integer=w527:u8)
          n232 = Build Array (concatenate)(w505, w527, w504, w525, w497) -> (w523:u8[])
          n233 = call "crc16-ccitt (x1021).vi"("unsigned byte array"=w523) -> ("CRC"=w522:u8[])  [unwired: 9 in, 1 out]
          n234 = Build Array (concatenate)(w524, w523, w522, w521) -> (w493:u8[])
          n235 = Byte Array To String(unsigned byte array=w497) -> (string=→"Send Array":string)
          n236 = call "GEA2 Add ESC Char.vi"("Message"=w493) -> ("Message Out"=w492:u8[])  [unwired: 14 in]
          n237 = local read "Enable Read ACK?"() -> (w495:bool)
          n238 = Array Size(array=w492) -> (size(s)=w517:i32)
          n239 = Byte Array To String(unsigned byte array=w492) -> (string=w494:string)
          n240 = VISA Write(VISA resource name=w531, write buffer=w494, error in (no error)=w515) -> (VISA resource name out=w520:refnum<visa-resource-name>, error out=w518:errorcluster)  [unwired: 1 out]
          n241 = Increment(x=w517) -> (x+1=w513:i32)
          n242 = Build Array (concatenate)(w492, w512) -> (w511:u8[])
          n243 = case shown="True" w495 {
            tunnel: w520 -> [_ w537]
            tunnel: [_ w536] -> w519
            tunnel: w518 -> [w532 w535]
            tunnel: w513 -> [_ w534]
            tunnel: [w532 w533] -> w498
            frame #0 {
            }
            frame #1 {
              n244 = VISA Read(VISA resource name=w537, byte count=w534, error in (no error)=w535) -> (read buffer=w536:string, error out=w533:errorcluster)  [unwired: 2 out]
            }
          }
          n245 = Byte Array To String(unsigned byte array=w511) -> (string=w516:string)
          n246 = Equal?(x=w498, y=w501) -> (x = y?=w499:bool)
          "Timeout ACK" <- w499
          n247 = Equal?(x=w516, y=w519) -> (x = y?=w503:bool)
          "ASCII ACK" <- w503
          n248 = case shown="True" w499 {
            tunnel: [w538 w541] -> w514
            tunnel: errorcluster {"status"=FALSE, "code"=0, "source"=""} ("Error Out") -> [_ w539]
            tunnel: w498 -> [w538 _]
            frame #0 {
            }
            frame #1 {
              n249 = call "Delay mS.vi"("Error In"=w539, "milliseconds to wait"=u32 10) -> ("Error Out"=w541:errorcluster)  [unwired: 13 in]
            }
          }
          "ASCII Count" <- w502
        }
        n250 = call <vilib>:"Add State(s) to Queue__jki_lib_state_machine.vi"("State(s) in (\"\")"=w491) -> ("States Out"=w490:string)  [unwired: 14 in]
      }
      frame #24 {
        n251 = Unbundle By Name(w543) -> ("ComPort"=w546:refnum<visa-resource-name>)
        n252 = for {
          N: 2 -> [_]
          tunnel: w546 -> [w583]
          tunnel: w545 -> [w567]
          tunnel: [w558] -> w544
          stop <- w559 stop-if-true
          w556 = errorcluster {"status"=TRUE, "code"=-1073807339, "source"="VISA Read in GEA2_ICP_Dryer_SM.vi"}  # timeout error
          w562 = T2 3 items=["CMD_Eval_Mode_Entry_CC1", "CMD_Eval_Mode_Entry_CC2", "CMD_Eval_Mode_Continue", "CMD_Send_DIAG_Info", "CMD_Enable_Debug_Log ", "CMD_Disable_Debug_Log ", "CMD_Send_Log_Data"] ("Command")
          w564 = u8 225  # ACK
          w573 = u8 227  # ETX
          w576 = u8 226  # STX
          n253 = call "Counter.vi"() -> ("Count"=→"Status Count":dbl)  [unwired: 11 in]
          n254 = call "Dryer_DSM_CMD.vi"("Command"=w562) -> ("CMD Array"=w577:u8[])  [unwired: 10 in]
          n255 = To Unsigned Byte Integer(number="Dryer Status 2 Send") -> (unsigned 8bit integer=w549:u8)
          n256 = Build Array(w549) -> (w551:u8[])
          n257 = Array Size(array=w577) -> (size(s)=w582:i32)
          n258 = Array Size(array=w551) -> (size(s)=w580:i32)
          n259 = local read "Source Address"() -> (w561:u8)
          n260 = local read "Destination Address"() -> (w560:u8)
          n261 = Compound Arithmetic op=ADD(7 ("x"), w582, w580) -> (w578:i32)
          n262 = To Unsigned Byte Integer(number=w578) -> (unsigned 8bit integer=w579:u8)
          n263 = Build Array (concatenate)(w561, w579, w560, w577, w551) -> (w575:u8[])
          n264 = call "crc16-ccitt (x1021).vi"("unsigned byte array"=w575) -> ("CRC"=w574:u8[])  [unwired: 9 in, 1 out]
          n265 = Build Array (concatenate)(w576, w575, w574, w573) -> (w565:u8[])
          n266 = for {
            tunnel: w583 -> [w601]
            tunnel: w567 -> [w600]
            tunnel: w565 -> [w599] mode=indexing
            tunnel: [w598] -> w572
            tunnel: [w596] -> w570
            n267 = Build Array(w599) -> (w595:u8[])
            n268 = Byte Array To String(unsigned byte array=w595) -> (string=w597:string)
            n269 = VISA Write(VISA resource name=w601, write buffer=w597, error in (no error)=w600) -> (VISA resource name out=w598:refnum<visa-resource-name>, error out=w596:errorcluster)  [unwired: 1 out]
          }
          n270 = Array Size(array=w565) -> (size(s)=w569:i32)
          n271 = Increment(x=w569) -> (x+1=w566:i32)
          n272 = Build Array (concatenate)(w565, w564) -> (w563:u8[])
          n273 = case shown="True" "Enable Read ACK?" {
            tunnel: w572 -> [_ w590]
            tunnel: ["" ("read buffer") w589] -> w571
            tunnel: w570 -> [w584 w588]
            tunnel: w566 -> [_ w587]
            tunnel: [w584 w586] -> w555
            frame #0 {
            }
            frame #1 {
              n274 = VISA Read(VISA resource name=w590, byte count=w587, error in (no error)=w588) -> (read buffer=w589:string, error out=w586:errorcluster)  [unwired: 2 out]
            }
          }
          n275 = Equal?(x=w555, y=w556) -> (x = y?=w554:bool)
          n276 = Byte Array To String(unsigned byte array=w563) -> (string=w568:string)
          n277 = case shown="False" w554 {
            tunnel: [w591 w594] -> w558
            tunnel: errorcluster {"status"=FALSE, "code"=0, "source"=""} ("Error Out") -> [_ w592]
            tunnel: w555 -> [w591 _]
            frame #0 {
            }
            frame #1 {
              n278 = call "Delay mS.vi"("Error In"=w592, "milliseconds to wait"=u32 10) -> ("Error Out"=w594:errorcluster)  [unwired: 13 in]
            }
          }
          n279 = Equal?(x=w568, y=w571) -> (x = y?=w559:bool)
          "STATUS ACK" <- w559
        }
        n280 = call <vilib>:"Add State(s) to Queue__jki_lib_state_machine.vi"("State(s) in (\"\")"=w548) -> ("States Out"=w547:string)  [unwired: 14 in]
      }
      frame #25 {
        w619 = u8 227  # ETX
        w625 = 7  # Header Length
        w622 = u8 226  # STX
        n281 = local read "Source Address"() -> (w607:u8)
        n282 = Unbundle By Name(w606) -> ("ComPort"=w626:refnum<visa-resource-name>)
        n283 = local read "Destination Address"() -> (w609:u8)
        n284 = Array Size(array="Sim Data") -> (size(s)=w605:i32)
        n285 = Compound Arithmetic op=ADD(w625, w605) -> (w623:i32)
        n286 = To Unsigned Byte Integer(number=w623) -> (unsigned 8bit integer=w624:u8)
        n287 = Build Array (concatenate)(w609, w624, w607, "Sim Data") -> (w621:u8[])
        n288 = call "crc16-ccitt (x1021).vi"("unsigned byte array"=w621) -> ("CRC"=w620:u8[])  [unwired: 9 in, 1 out]
        n289 = Build Array (concatenate)(w622, w621, w620, w619) -> (w602:u8[])
        n290 = local write "Command Bytes"(w602) -> ()
        n291 = flat-sequence {
          tunnel: [w636] -> w604
          tunnel: w613 -> [_]
          frame #0 {
            n292 = Tick Count (ms)() -> (millisecond timer value=w636:u32)
          }
        }
        n293 = local write "tStart"(w604) -> ()
        n294 = for {
          tunnel: w626 -> [w635]
          tunnel: w613 -> [w634]
          tunnel: w602 -> [w633] mode=indexing
          tunnel: [w632] -> w618
          tunnel: [w630] -> w616
          tunnel: w604 -> [_]
          n295 = Build Array(w633) -> (w629:u8[])
          n296 = Byte Array To String(unsigned byte array=w629) -> (string=w631:string)
          n297 = VISA Write(VISA resource name=w635, write buffer=w631, error in (no error)=w634) -> (VISA resource name out=w632:refnum<visa-resource-name>, error out=w630:errorcluster)  [unwired: 1 out]
        }
        n298 = Array Size(array=w602) -> (size(s)=w615:i32)
        n299 = Byte Array To String(unsigned byte array=w602) -> (string=w614:string)
        n300 = VISA Read(VISA resource name=w618, byte count=w615, error in (no error)=w616) -> (read buffer=w617:string, error out=w612:errorcluster)  [unwired: 2 out]
        n301 = Equal?(x=w614, y=w617) -> (x = y?=w603:bool)
        n302 = call "Delay mS.vi"("Error In"=w612, "milliseconds to wait"=u32 10) -> ("Error Out"=w611:errorcluster)  [unwired: 13 in]
        n303 = local write "WriteOK"(w603) -> ()
        n304 = call <vilib>:"Add State(s) to Queue__jki_lib_state_machine.vi"("State(s) in (\"\")"=w628) -> ("States Out"=w627:string)  [unwired: 14 in]
      }
      frame #26 {
        w639 = u32 8  # Idle Time
        w649 = -1073807252  # Buffer Overflow
        w657 = errorcluster {"status"=TRUE, "code"=-1073807339, "source"="VISA Read in GEA2_ICP_Dryer_SM.vi"}  # timeout error
        # "Try to make sure not in mid of transmission"
        # "If there is data, initialize serial data in."
        # "Read the port:"
        n305 = Unbundle By Name(w660) -> ("ComPort"=w641:refnum<visa-resource-name>)
        n306 = call "GEA2 Wait for Bus Idle.vi"("Error In"=w643, "Idle Time"=w639, "ComPort"=w641) -> ("error out"=w642:errorcluster, "Bytes at Port"=w640:u32)  [unwired: 7 in]
        "Bytes At Port" <- w640
        n307 = To Long Integer(number=w640) -> (32bit integer=w637:i32)
        n308 = VISA Read(VISA resource name=w641, byte count=w640, error in (no error)=w642) -> (read buffer=w659:string, error out=w650:errorcluster)  [unwired: 2 out]
        "read buffer" <- w659
        n309 = Unbundle By Name(w650) -> ("code"=w648:i32)
        n310 = String To Byte Array(string=w659) -> (unsigned byte array=w658:u8[])
        "ReadArray" <- w658
        n311 = Equal?(x=w650, y=w657) -> (x = y?=w656:bool)
        "Timeout" <- w656
        n312 = Equal?(x=w648, y=w649) -> (x = y?=w651:bool)
        n313 = Bundle By Name(cluster=w660, "Total Bytes Read"=w637, "ReadArray"=w658, "CRCArray"=u8[] [] ("ReadArray"), "Current Read Index"=0) -> (w654:T9)
        n314 = Or(x=w656, y=w651) -> (x .or. y?=w652:bool)
        n315 = case shown="True" w652 {
          tunnel: [w666 w667] -> w646
          tunnel: errorcluster {"status"=FALSE, "code"=0, "source"=""} ("Error Out") -> [_ w667]
          tunnel: w650 -> [w666 _]
          frame #0 {
          }
          frame #1 {
          }
        }
        n316 = Bundle By Name(cluster=w654, "Dryer Status Serial Data In.Command:Data"="") -> (w653:T9)
        n317 = disable-structure shown="Enabled" {
          disable-tunnel: w646 -> [w664 _]
          frame #0 {
            n318 = call <vilib>:"Simple Error Handler.vi"("error in (no error)"=w664) -> ()  [unwired: 4 in, 5 out]
          }
          frame #1 {
          }
        }
        n319 = local read "Exit"() -> (w645:bool)
        n320 = case shown="False" w645 {
          tunnel: [_ "Exit" ("State(s) in Front (\"\")")] -> w644
          frame #0 {
          }
          frame #1 {
          }
        }
        n321 = call <vilib>:"Add State(s) to Queue__jki_lib_state_machine.vi"("State(s) in Front (\"\")"=w644, "State(s) in (\"\")"=w663) -> ("States Out"=w662:string)  [unwired: 13 in]
      }
      frame #27 {
        # "Template Separator\n(You can make a copy of, or modify, this frame)"
        n322 = call <vilib>:"Add State(s) to Queue__jki_lib_state_machine.vi"("State(s) in (\"\")"=w671) -> ("States Out"=w670:string)  [unwired: 14 in]
      }
      frame #28 {
        # "Template Separator\n(You can make a copy of, or modify, this frame)"
        n323 = disable-structure shown="Enabled" {
          disable-tunnel: w673 -> [w682 w685]
          disable-tunnel: [w680 w683] -> w675
          frame #0 {
            n324 = Unbundle By Name(w682) -> ("ReadArray"=w681:u8[])
            n325 = Array Size(array=w681) -> (size(s)=w680:i32)
          }
          frame #1 {
            n326 = Unbundle By Name(w685) -> ("Total Bytes Read"=w684:i32)
            n327 = To Long Integer(number=w684) -> (32bit integer=w683:i32)
          }
        }
        n328 = Equal To 0?(x=w675) -> (x = 0?=w674:bool)
        n329 = case shown="True" w674 {
          tunnel: ["Interpret Bytes" ("State(s) in Front (\"\")") "Parse: STX\nParse: Destination\nParse: Length\nParse: Source\nParse: Bytes Data\nParse: CRC1\nParse: CRC2\nCheckCRC\nParse: ETX\nInterpret Bytes\nCheck Complete" ("State(s) in Front (\"\")")] -> w676
          tunnel: w673 -> [w688 w690]
          tunnel: [w687 w690] -> w672
          frame #0 {
            n330 = Bundle By Name(cluster=w688, "Bytes Data"=u8[] []) -> (w687:T9)
          }
          frame #1 {
          }
        }
        n331 = call <vilib>:"Add State(s) to Queue__jki_lib_state_machine.vi"("State(s) in Front (\"\")"=w676, "State(s) in (\"\")"=w679) -> ("States Out"=w678:string)  [unwired: 13 in]
      }
      frame #29 {
        # "Your code here.\n(You can make a copy of, or modify, this frame)"
        n332 = Unbundle By Name(w702) -> ("Total Bytes Read"=w693:i32, "Current Read Index"=w694:i32, "ReadArray"=w697:u8[])
        "Current Read Index" <- w694
        n333 = while {
          tunnel: [w710] -> w700
          tunnel: w693 -> [w709]
          shift-right: [w706] -> w692
          shift-left: w694 -> [w707]
          tunnel: w697 -> [w713]
          stop <- w711 stop-if-true
          w705 = u8 226  # STX
          n334 = Increment(x=w707) -> (x+1=w706:i32)
          n335 = Index Array(array=w713, index=w707) -> (element=w712:u8)
          n336 = Less?(x=w709, y=w706) -> (x < y?=w708:bool)
          n337 = Equal?(x=w712, y=w705) -> (x = y?=w710:bool)
          n338 = Or(x=w708, y=w710) -> (x .or. y?=w711:bool)
        }
        n339 = case shown="False" w700 {
          tunnel: w696 -> [w717 w725]
          tunnel: [w715 w725] -> w699
          tunnel: ["Exit" ("State(s) in Front (\"\")") _] -> w698
          frame #0 {
            n340 = disable-structure shown="Enabled" {
              disable-tunnel: w717 -> [w720 w724]
              disable-tunnel: [w718 w724] -> _
              disable-tunnel: [_ w723] -> w715
              frame #0 {
                n341 = call "Error Bool Enumerator.vi"("Error Enum"=HEWH_Error_Enumeration."GEA2 STX", "Error In"=w720, "Error?"=TRUE) -> ("Error Out"=w718:errorcluster)  [unwired: 6 in]
              }
              frame #1 {
                # "Partial Message"
                n342 = Bundle By Name(cluster=w724, "source"="Partial GEA Message") -> (w723:errorcluster)
              }
            }
            n343 = local write "Partial Message"(TRUE ("Partial Message")) -> ()
          }
          frame #1 {
          }
        }
        n344 = Bundle By Name(cluster=w702, "Current Read Index"=w692, "Bytes Data"=u8[] []) -> (w701:T9)
        n345 = call <vilib>:"Add State(s) to Queue__jki_lib_state_machine.vi"("State(s) in Front (\"\")"=w698, "State(s) in (\"\")"=w704) -> ("States Out"=w703:string)  [unwired: 13 in]
      }
      frame #30 {
        w736 = u8 224  # ESC
        n346 = Unbundle By Name(w738) -> ("CRCArray"=w733:u8[], "ReadArray"=w729:u8[], "Current Read Index"=w731:i32)  [unwired: 1 out]
        n347 = Increment(x=w731) -> (x+1=w728:i32)
        n348 = Index Array(array=w729, index=w731) -> (element=w730:u8)
        n349 = Equal?(x=w730, y=w736) -> (x = y?=w735:bool)
        n350 = case shown="True" w735 {
          tunnel: [w742 w745] -> w726
          tunnel: [w741 w743] -> w727
          tunnel: w729 -> [_ w746]
          tunnel: w730 -> [w742 _]
          tunnel: w728 -> [w741 w744]
          frame #0 {
          }
          frame #1 {
            n351 = Increment(x=w744) -> (x+1=w743:i32)
            n352 = Index Array(array=w746, index=w744) -> (element=w745:u8)
          }
        }
        "Source Read" <- w726
        n353 = Build Array (concatenate)(w733, w726) -> (w732:u8[])
        n354 = Bundle By Name(cluster=w738, "CRCArray"=w732, "Current Read Index"=w727) -> (w737:T9)
        n355 = call <vilib>:"Add State(s) to Queue__jki_lib_state_machine.vi"("State(s) in (\"\")"=w740) -> ("States Out"=w739:string)  [unwired: 14 in]
      }
      frame #31 {
        w769 = -3  # CRC + ETX
        w757 = u8 224  # ESC
        n356 = Unbundle By Name(w775) -> ("Total Bytes Read"=w764:i32, "ReadArray"=w750:u8[], "CRCArray"=w770:u8[], "Current Read Index"=w749:i32)  [unwired: 1 out]
        n357 = Increment(x=w749) -> (x+1=w766:i32)
        n358 = Index Array(array=w750, index=w749) -> (element=w765:u8)
        n359 = Equal?(x=w765, y=w757) -> (x = y?=w773:bool)
        n360 = case shown="True" w773 {
          tunnel: [w782 w784] -> w748
          tunnel: [w783 w785] -> w762
          tunnel: w750 -> [_ _]
          tunnel: w750 -> [_ w787]
          tunnel: w766 -> [w783 w786]
          tunnel: w765 -> [w782 _]
          frame #0 {
          }
          frame #1 {
            n361 = Index Array(array=w787, index=w786) -> (element=w784:u8)
            n362 = Increment(x=w786) -> (x+1=w785:i32)
          }
        }
        "Length" <- w748
        n363 = Array Subset(array=w750, index=w749, length=w748) -> (w747:u8[])
        n364 = Equal?(x=w747, y=w757) -> (x = y?=w756:bool[])
        n365 = Boolean To (0,1)(Boolean=w756) -> (0, 1=w755:i16[])
        n366 = Add Array Elements(numeric array=w755) -> (sum=w754:i16)
        n367 = Multiply(x=w754, y=i16 -1) -> (x*y=w752:i16)
        n368 = To Long Integer(number=w752) -> (32bit integer=w751:i32)
        n369 = Build Array (concatenate)(w770, w748) -> (w771:u8[])
        n370 = To Long Integer(number=w748) -> (32bit integer=w761:i32)
        n371 = Bundle By Name(cluster=w775, "Current Read Index"=w762, "CRCArray"=w771, "Bytes Remaining"=w748) -> (w774:T9)
        n372 = Compound Arithmetic op=ADD(w762, w769, w761, w751) -> (w768:i32)
        n373 = To Long Integer(number=w768) -> (32bit integer=w763:i32)
        n374 = Less?(x=w764, y=w763) -> (x < y?=w767:bool)
        "Partial Message" <- w767
        n375 = local read "Mode"() -> (w760:T5)
        n376 = case shown="True" w767 {
          tunnel: w760 -> [_ w779]
          tunnel: [w777 w778] -> w758
          tunnel: w759 -> [w777 _]
          frame #0 {
          }
          frame #1 {
            n377 = case shown="\"Read Continuous\"" w779 {
              tunnel: ["Exit" ("State(s) in Front (\"\")") "Read Continue" ("State(s) in Front (\"\")")] -> w778
              frame #0 {
              }
              frame #1 {
              }
            }
          }
        }
        n378 = call <vilib>:"Add State(s) to Queue__jki_lib_state_machine.vi"("State(s) in (\"\")"=w758) -> ("States Out"=w776:string)  [unwired: 14 in]
      }
      frame #32 {
        w797 = u8 224  # ESC
        n379 = Unbundle By Name(w801) -> ("ReadArray"=w788:u8[], "Current Read Index"=w793:i32)
        n380 = Increment(x=w793) -> (x+1=w792:i32)
        n381 = Index Array(array=w788, index=w793) -> (element=w789:u8)
        n382 = Equal?(x=w789, y=w797) -> (x = y?=w796:bool)
        n383 = case shown="True" w796 {
          tunnel: [w805 w806] -> w791
          tunnel: [w804 w808] -> w794
          tunnel: w788 -> [_ w809]
          tunnel: w792 -> [w804 w807]
          tunnel: w789 -> [w805 _]
          frame #0 {
          }
          frame #1 {
            n384 = Index Array(array=w809, index=w807) -> (element=w806:u8)
            n385 = Increment(x=w807) -> (x+1=w808:i32)
          }
        }
        "Destination Read" <- w791
        n386 = local read "Source Address"() -> (w798:u8)
        n387 = Build Array(w791) -> (w790:u8[])
        n388 = Bundle By Name(cluster=w801, "Current Read Index"=w794, "CRCArray"=w790) -> (w800:T9)
        n389 = Equal?(x=w791, y=w798) -> (x = y?=→"Message for Me":bool)
        n390 = call <vilib>:"Add State(s) to Queue__jki_lib_state_machine.vi"("State(s) in (\"\")"=w803) -> ("States Out"=w802:string)  [unwired: 14 in]
      }
      frame #33 {
        w828 = u8 224  # ESC
        n391 = Unbundle By Name(w830) -> ("ReadArray"=w813:u8[], "CRCArray"=w824:u8[], "Bytes Remaining"=w823:u8, "Bytes Data"=w821:u8[], "Current Read Index"=w812:i32)
        n392 = Increment(x=w812) -> (x+1=w811:i32)
        n393 = Index Array(array=w813, index=w812) -> (element=w810:u8)
        n394 = Equal?(x=w810, y=w828) -> (x = y?=w827:bool)
        n395 = case shown="True" w827 {
          tunnel: [w834 w836] -> w819
          tunnel: [w835 w839] -> w822
          tunnel: w813 -> [_ w838]
          tunnel: w813 -> [_ _]
          tunnel: w811 -> [w835 w837]
          tunnel: w810 -> [w834 _]
          frame #0 {
          }
          frame #1 {
            n396 = Index Array(array=w838, index=w837) -> (element=w836:u8)
            n397 = Increment(x=w837) -> (x+1=w839:i32)
          }
        }
        n398 = Decrement(x=w823) -> (x-1=w816:u8)
        n399 = Build Array (concatenate)(w821, w819) -> (w820:u8[])
        n400 = Build Array (concatenate)(w824, w819) -> (w825:u8[])
        n401 = Subtract(x=w816, y=u8 7) -> (x-y=w814:u8)
        n402 = Bundle By Name(cluster=w830, "Current Read Index"=w822, "CRCArray"=w825, "Bytes Remaining"=w816, "Bytes Data"=w820) -> (w829:T9)
        n403 = Greater Than 0?(x=w814) -> (x > 0?=w818:bool)
        n404 = case shown="True" w818 {
          tunnel: [_ "Parse: Bytes Data" ("State(s) in Front (\"\")")] -> w817
          frame #0 {
          }
          frame #1 {
          }
        }
        n405 = call <vilib>:"Add State(s) to Queue__jki_lib_state_machine.vi"("State(s) in Front (\"\")"=w817, "State(s) in (\"\")"=w832) -> ("States Out"=w831:string)  [unwired: 13 in]
      }
      frame #34 {
        w849 = u8 224  # ESC
        n406 = Unbundle By Name(w851) -> ("ReadArray"=w844:u8[], "Current Read Index"=w843:i32)  [unwired: 1 out]
        n407 = Increment(x=w843) -> (x+1=w842:i32)
        n408 = Index Array(array=w844, index=w843) -> (element=w841:u8)
        n409 = Equal?(x=w841, y=w849) -> (x = y?=w848:bool)
        n410 = case shown="True" w848 {
          tunnel: [w854 w856] -> w845
          tunnel: [w855 w859] -> w846
          tunnel: w844 -> [_ w858]
          tunnel: w842 -> [w855 w857]
          tunnel: w841 -> [w854 _]
          frame #0 {
          }
          frame #1 {
            n411 = Index Array(array=w858, index=w857) -> (element=w856:u8)
            n412 = Increment(x=w857) -> (x+1=w859:i32)
          }
        }
        n413 = Build Array(w845) -> (w840:u8[])
        n414 = Bundle By Name(cluster=w851, "Current Read Index"=w846, "CRCRead"=w840) -> (w850:T9)
        n415 = call <vilib>:"Add State(s) to Queue__jki_lib_state_machine.vi"("State(s) in (\"\")"=w853) -> ("States Out"=w852:string)  [unwired: 14 in]
      }
      frame #35 {
        w870 = u8 224  # ESC
        n416 = Unbundle By Name(w872) -> ("ReadArray"=w861:u8[], "CRCRead"=w864:u8[], "Current Read Index"=w863:i32)
        n417 = Increment(x=w863) -> (x+1=w862:i32)
        n418 = Index Array(array=w861, index=w863) -> (element=w860:u8)
        n419 = Equal?(x=w860, y=w870) -> (x = y?=w869:bool)
        n420 = case shown="True" w869 {
          tunnel: [w875 w877] -> w866
          tunnel: [w876 w880] -> w867
          tunnel: w861 -> [_ w879]
          tunnel: w862 -> [w876 w878]
          tunnel: w860 -> [w875 _]
          frame #0 {
          }
          frame #1 {
            n421 = Increment(x=w878) -> (x+1=w880:i32)
            n422 = Index Array(array=w879, index=w878) -> (element=w877:u8)
          }
        }
        n423 = Build Array (concatenate)(w864, w866) -> (w865:u8[])
        n424 = Bundle By Name(cluster=w872, "Current Read Index"=w867, "CRCRead"=w865) -> (w871:T9)
        n425 = call <vilib>:"Add State(s) to Queue__jki_lib_state_machine.vi"("State(s) in (\"\")"=w874) -> ("States Out"=w873:string)  [unwired: 14 in]
      }
      frame #36 {
        # "Your code here.\n(You can make a copy of, or modify, this frame)"
        n426 = Unbundle By Name(w885) -> ("CRCRead"=w882:u8[], "CRCArray"=w887:u8[])
        "CRCRead" <- w882
        "CRCArray" <- w887
        n427 = call "crc16-ccitt (x1021).vi"("error in (no error)"=w888, "unsigned byte array"=w887) -> ("error out (dup)"=w883:errorcluster, "CRC"=w886:u8[])  [unwired: 8 in]
        "CRC Calc" <- w886
        n428 = Equal?(x=w882, y=w886) -> (x = y?=w881:bool)
        "CRC Match" <- w881
        n429 = Bundle By Name(cluster=w885, "CRC"=w881) -> (w884:T9)
        n430 = call <vilib>:"Add State(s) to Queue__jki_lib_state_machine.vi"("State(s) in (\"\")"=w890) -> ("States Out"=w889:string)  [unwired: 14 in]
      }
      frame #37 {
        w891 = u8 227  # ETX
        # "Your code here.\n(You can make a copy of, or modify, this frame)"
        n431 = Unbundle By Name(w901) -> ("ReadArray"=w896:u8[], "Current Read Index"=w892:i32)
        n432 = Index Array(array=w896, index=w892) -> (element=w894:u8)
        n433 = Increment(x=w892) -> (x+1=w893:i32)
        n434 = Equal?(x=w894, y=w891) -> (x = y?=w899:bool)
        n435 = case shown="False" w899 {
          tunnel: w895 -> [w907 w909]
          tunnel: [w904 w909] -> w898
          tunnel: ["Exit" ("State(s) in Front (\"\")") _] -> w897
          frame #0 {
            n436 = call "Error Bool Enumerator.vi"("Error Enum"=HEWH_Error_Enumeration."GEA2 ETX", "Error In"=w907, "Error?"=TRUE) -> ("Error Out"=w904:errorcluster)  [unwired: 6 in]
          }
          frame #1 {
          }
        }
        n437 = Bundle By Name(cluster=w901, "Current Read Index"=w893) -> (w900:T9)
        n438 = call <vilib>:"Add State(s) to Queue__jki_lib_state_machine.vi"("State(s) in Front (\"\")"=w897, "State(s) in (\"\")"=w903) -> ("States Out"=w902:string)  [unwired: 13 in]
      }
      frame #38 {
        n439 = Unbundle By Name(w911) -> ("ComPort"=w913:refnum<visa-resource-name>, "CRC"=w910:bool)
        n440 = case shown="True" w910 {
          tunnel: w914 -> [w917 w926]
          tunnel: w913 -> [_ w920]
          tunnel: [w917 w919] -> w912
          frame #0 {
          }
          frame #1 {
            w921 = u8 225  # ACK
            n441 = Build Array(w921) -> (w924:u8[])
            n442 = Byte Array To String(unsigned byte array=w924) -> (string=w923:string)
            n443 = VISA Write(VISA resource name=w920, write buffer=w923, error in (no error)=w926) -> (VISA resource name out=w925:refnum<visa-resource-name>, error out=w922:errorcluster)  [unwired: 1 out]
            n444 = case shown="True" TRUE {
              tunnel: w925 -> [_ w938]
              tunnel: w923 -> [_ w936]
              tunnel: w922 -> [w927 w935]
              tunnel: [w927 w929] -> w919
              frame #0 {
                # "Skip Readback"
              }
              frame #1 {
                n445 = VISA Read(VISA resource name=w938, byte count=u32 1, error in (no error)=w935) -> (read buffer=w933:string, error out=w934:errorcluster)  [unwired: 2 out]
                n446 = Equal?(x=w936, y=w933) -> (x = y?=w931:bool)
                "Read_ACK" <- w931
                n447 = String To Byte Array(string=w933) -> (unsigned byte array=→"ACK(E1?)":u8[])
                n448 = Not(x=w931) -> (.not. x?=w930:bool)
                n449 = call "Error Bool Enumerator.vi"("Error Enum"=HEWH_Error_Enumeration."GEA2 Send ACK Mismatch", "Error In"=w934, "Error?"=w930) -> ("Error Out"=w929:errorcluster)  [unwired: 6 in]
              }
            }
          }
        }
        n450 = call <vilib>:"Add State(s) to Queue__jki_lib_state_machine.vi"("State(s) in (\"\")"=w916) -> ("States Out"=w915:string)  [unwired: 14 in]
      }
      frame #39 {
        w941 = FALSE  # Fault Cond Detected
        # "Template Separator\n(You can make a copy of, or modify, this frame)"
        n451 = Unbundle By Name(w946) -> ("Bytes Data"=w949:u8[], "ComPort"=w942:refnum<visa-resource-name>, "Dryer Status Serial Data In"=w948:T3)
        "DataReturned" <- w949
        n452 = call "Get Com Number.vi"("ComPort Local Copy"=w942) -> ("Com Num"=w947:u8)  [unwired: 10 in]
        n453 = global read "Globals Wilt.vi" "Bad Com Limit"() -> (w940:i32)
        n454 = To Unsigned Long Integer(number=w940) -> (unsigned 32bit integer=w939:u32)
        n455 = call "Dryer Status.vi"("Bytes Comm"=w949, "Fault Cond Detected"=w941, "Dryer Status Serial Data In"=w948, "Com Port"=w947, "Err Count Lim"=w939) -> ("Dryer Status Serial Data Out"=w943:T3)  [unwired: 10 in]
        "Dryer Status Serial Data Out" <- w943
        n456 = Unbundle By Name(w943) -> ("Command:Data"=→"Com:Data":string)
        n457 = Bundle By Name(cluster=w946, "Dryer Status Serial Data In"=w943) -> (w945:T9)
        n458 = call <vilib>:"Add State(s) to Queue__jki_lib_state_machine.vi"("State(s) in (\"\")"=w952) -> ("States Out"=w951:string)  [unwired: 14 in]
      }
      frame #40 {
        # "Template Separator\n(You can make a copy of, or modify, this frame)"
        n459 = Unbundle By Name(w955) -> ("Total Bytes Read"=w959:i32, "Current Read Index"=w958:i32, "Reset MSG Count"=w956:bool)
        n460 = Subtract(x=w959, y=w958) -> (x-y=w957:i32)
        n461 = call "Counter.vi"("Reset"=w956) -> ("Count"=→"Num Messages":dbl)  [unwired: 10 in]
        n462 = Greater?(x=w957, y=7) -> (0:w962:bool)
        n463 = case shown="True" w962 {
          tunnel: [_ "Parse: STX\nParse: Destination\nParse: Length\nParse: Source\nParse: Bytes Data\nParse: CRC1\nParse: CRC2\nCheckCRC\nParse: ETX\nInterpret Bytes\nCheck Complete" ("State(s) in Front (\"\")")] -> w961
          frame #0 {
          }
          frame #1 {
          }
        }
        n464 = Bundle By Name(cluster=w955, "Reset MSG Count"=FALSE) -> (w954:T9)
        n465 = call <vilib>:"Add State(s) to Queue__jki_lib_state_machine.vi"("State(s) in Front (\"\")"=w961, "State(s) in (\"\")"=w966) -> ("States Out"=w965:string)  [unwired: 13 in]
      }
      frame #41 {
        # "Template Separator\n(You can make a copy of, or modify, this frame)"
        n466 = local read "Com:Data"() -> (w985:string)
        n467 = local read "Bytes At Port"() -> (w980:u32)
        n468 = Unbundle By Name(w973) -> ("Reset Pulse"=w972:bool)
        n469 = Search and Replace String(input string=w985, search string="No Com", replace string="" ("replace string (\"\")")) -> (result string=w982:string)  [unwired: 5 in, 3 out]
        n470 = To Long Integer(number=w980) -> (32bit integer=w976:i32)
        n471 = To Long Integer(number=u32 7 ("y")) -> (32bit integer=w975:i32)
        n472 = call <vilib>:"Trim Whitespace.vi"("string"=w982) -> ("trimmed string"=w981:string)  [unwired: 1 in]
        n473 = Subtract(x=w976, y=w975) -> (x-y=w978:i32)
        n474 = Greater Than 0?(x=w978) -> (x > 0?=w977:bool)
        n475 = call "Counter.vi"("Reset"=w972) -> ("Count"=→"Read Pulse":dbl)  [unwired: 10 in]
        n476 = case shown="True" w977 {
          tunnel: w981 -> [_ w1000]
          tunnel: [w996 w997] -> w987
          frame #0 {
            n477 = local read "Com:Data Buffer"() -> (w996:string)
          }
          frame #1 {
            n478 = local read "Com:Data Buffer"() -> (w998:string)
            n479 = Concatenate Strings(w1000, "\n", w998) -> (w997:string)
            n480 = local write "Com:Data Buffer"(w997) -> ()
          }
        }
        n481 = flat-sequence {
          tunnel: ["ReadData\nData: Parse\nRead Continue"] -> w970
          tunnel: w987 -> [w994]
          frame #0 {
            n482 = local write "Com:Data"(w994) -> ()
            n483 = Wait (ms)(milliseconds to wait=u32 2000) -> ()  [unwired: 1 out]
          }
        }
        n484 = Bundle By Name(cluster=w973, "Reset Pulse"=FALSE ("Reset MSG Count"), "Dryer Status Serial Data In.Command:Data"="") -> (w989:T9)
        n485 = local read "Exit"() -> (w971:bool)
        n486 = Select(t="Exit", s=w971, f=w970) -> (s? t:f=w968:string)
        n487 = call <vilib>:"Add State(s) to Queue__jki_lib_state_machine.vi"("State(s) in Front (\"\")"=w968, "State(s) in (\"\")"=w992) -> ("States Out"=w991:string)  [unwired: 13 in]
      }
      frame #42 {
        # "Template Separator\n(You can make a copy of, or modify, this frame)"
        n488 = call <vilib>:"Add State(s) to Queue__jki_lib_state_machine.vi"("State(s) in (\"\")"=w1004) -> ("States Out"=w1003:string)  [unwired: 14 in]
      }
      frame #43 {
        # "Template Separator\n(You can make a copy of, or modify, this frame)"
        n489 = call <vilib>:"Add State(s) to Queue__jki_lib_state_machine.vi"("State(s) in Front (\"\")"="Wait for Initialization\nWait for Start\nTimed Dry\nWait for Restart", "State(s) in (\"\")"=w1009) -> ("States Out"=w1008:string)  [unwired: 13 in]
      }
      frame #44 {
        w1010 = FALSE ("CRC")
        w1027 = T2 4 items=["CMD_Eval_Mode_Entry_CC1", "CMD_Eval_Mode_Entry_CC2", "CMD_Eval_Mode_Continue", "CMD_Send_DIAG_Info", "CMD_Enable_Debug_Log ", "CMD_Disable_Debug_Log ", "CMD_Send_Log_Data"] ("Dryer Cmd")
        w1028 = T2 1 items=["CMD_Eval_Mode_Entry_CC1", "CMD_Eval_Mode_Entry_CC2", "CMD_Eval_Mode_Continue", "CMD_Send_DIAG_Info", "CMD_Enable_Debug_Log ", "CMD_Disable_Debug_Log ", "CMD_Send_Log_Data"] ("Dryer Cmd")
        # "Template Separator\n(You can make a copy of, or modify, this frame)"
        n490 = Unbundle By Name(w1017) -> ("ReadCM1Flag"=w1021:bool, "ReadCM2Flag"=w1019:bool)
        n491 = local read "Com:Data"() -> (w1023:string)
        n492 = call "Type Conv - Dryer Cmd to String.vi"("Dryer Cmd"=w1028) -> ("Read String"=w1026:string)  [unwired: 10 in]
        n493 = call "Type Conv - Dryer Cmd to String.vi"("Dryer Cmd"=w1027) -> ("Read String"=w1024:string)  [unwired: 10 in]
        n494 = xnode "Match Regular Expression"("input string"=w1023, "regular expression"=w1026) -> ("offset past match"=w1029:i32)  [unwired: 4 in, 4 out]
        n495 = Greater Or Equal To 0?(x=w1029) -> (x >= 0?=w1022:bool)
        n496 = xnode "Match Regular Expression"("input string"=w1023, "regular expression"=w1024) -> ("offset past match"=w1025:i32)  [unwired: 4 in, 4 out]
        n497 = Greater Or Equal To 0?(x=w1025) -> (x >= 0?=w1020:bool)
        n498 = local write "CRC Match"(w1010) -> ()
        n499 = Or(x=w1021, y=w1022) -> (x .or. y?=w1012:bool)
        "ReadCM1Flag" <- w1012
        n500 = Or(x=w1019, y=w1020) -> (x .or. y?=w1011:bool)
        "ReadCM2Flag" <- w1011
        n501 = Bundle By Name(cluster=w1017, "Dryer Status Serial Data In.Command:Data"="", "CRC"=w1010, "ReadCM1Flag"=w1012, "ReadCM2Flag"=w1011) -> (w1015:T9)
        n502 = And(x=w1012, y=w1011) -> (x .and. y?=w1018:bool)
        "Sim Init" <- w1018
        n503 = case shown="False" w1018 {
          tunnel: ["ReadData\nData: Parse\nSendACK\nWait for Initialization" "Send Status"] -> w1030
          tunnel: w1015 -> [w1034 w1036]
          tunnel: [w1034 w1036] -> w1014
          frame #0 {
          }
          frame #1 {
            n504 = local write "Dryer Status 2 Send"(Dryer_Status_Ctrl."Eval Mode Entered" ("Dryer Status 2 Send")) -> ()
          }
        }
        n505 = Wait Until Next ms Multiple(millisecond multiple=u32 150) -> ()  [unwired: 1 out]
        n506 = call <vilib>:"Add State(s) to Queue__jki_lib_state_machine.vi"("State(s) in Front (\"\")"=w1030, "State(s) in (\"\")"=w1033) -> ("States Out"=w1032:string)  [unwired: 13 in]
      }
      frame #45 {
        # "Template Separator\n(You can make a copy of, or modify, this frame)"
        n507 = local read "Period of STATUS (Counts)"() -> (w1261:dbl)
        n508 = call "Counter.vi"() -> ("Count"=w1260:dbl)  [unwired: 11 in]
        n509 = Quotient & Remainder(x=w1260, y=w1261) -> (x-y*floor(x/y)=w1259:dbl)  [unwired: 1 out]
        n510 = Equal To 0?(x=w1259) -> (x = 0?=w1258:bool)
        n511 = Select(t="Send Status\n", s=w1258, f="") -> (s? t:f=w1253:string)
        n512 = case shown="True" "Sim Dryer Start" {
          selector: "Sim Dryer Start" -> [_ w1270]
          tunnel: ["Wait for Start" ""] -> w1255
          frame #0 {
          }
          frame #1 {
            n513 = call "E-Time.vi"() -> ("Elapsed Time (sec)"=→"Tstart":dbl)  [unwired: 9 in, 2 out]
            n514 = local write "Sim Dryer Start"(FALSE ("Sim Dryer Start")) -> ()
            "Start Pressed" <- w1270
          }
        }
        n515 = Concatenate Strings(w1253, w1255) -> (w1254:string)
        n516 = Wait Until Next ms Multiple(millisecond multiple=u32 1000) -> ()  [unwired: 1 out]
        n517 = call <vilib>:"Add State(s) to Queue__jki_lib_state_machine.vi"("State(s) in Front (\"\")"=w1254, "State(s) in (\"\")"=w1267) -> ("States Out"=w1266:string)  [unwired: 13 in]
      }
      frame #46 {
        # "Template Separator\n(You can make a copy of, or modify, this frame)"
        n518 = flat-sequence {
          tunnel: [w1293] -> w1278
          tunnel: [w1288] -> w1277
          frame #0 {
            n519 = local write "Dryer Status 2 Send"(Dryer_Status_Ctrl."Cycle Running" ("Dryer Status 2 Send")) -> ()
            n520 = local read "Period of STATUS (Counts)"() -> (w1291:dbl)
            n521 = local read "Tstart"() -> (w1297:dbl)
            n522 = call "E-Time.vi"() -> ("Elapsed Time (sec)"=w1298:dbl)  [unwired: 9 in, 2 out]
            n523 = Subtract(x=w1298, y=w1297) -> (x-y=w1295:dbl)
            n524 = call "Counter.vi"() -> ("Count"=w1290:dbl)  [unwired: 11 in]
            n525 = Subtract(x=w1295, y="Cycle Time (s)") -> (x-y=w1294:dbl)
            "Time Left" <- w1294
            n526 = Greater Than 0?(x=w1294) -> (x > 0?=w1293:bool)
            n527 = Quotient & Remainder(x=w1290, y=w1291) -> (x-y*floor(x/y)=w1289:dbl)  [unwired: 1 out]
            n528 = Equal To 0?(x=w1289) -> (x = 0?=w1287:bool)
            n529 = Select(t="Send Status\nSend ASCII\nTimed Dry", s=w1287, f="Send ASCII\nTimed Dry") -> (s? t:f=w1288:string)
            "Drying" <- TRUE
          }
        }
        n530 = case shown="False" w1278 {
          tunnel: [w1300 ""] -> w1281
          tunnel: w1277 -> [w1300 _]
          frame #0 {
          }
          frame #1 {
            n531 = local write "Drying"(FALSE ("Drying")) -> ()
          }
        }
        n532 = local read "Exit"() -> (w1274:bool)
        n533 = Wait Until Next ms Multiple(millisecond multiple=u32 1000) -> ()  [unwired: 1 out]
        n534 = case shown="True" w1274 {
          tunnel: [_ "Exit"] -> w1273
          frame #0 {
          }
          frame #1 {
          }
        }
        n535 = call <vilib>:"Add State(s) to Queue__jki_lib_state_machine.vi"("State(s) in Front (\"\")"=w1281, "State(s) in (\"\")"=w1283) -> ("States Out"=w1276:string)  [unwired: 13 in]
        n536 = call <vilib>:"Add State(s) to Queue__jki_lib_state_machine.vi"("State(s) in Front (\"\")"=w1273, "State(s) in (\"\")"=w1276) -> ("States Out"=w1275:string)  [unwired: 13 in]
      }
      frame #47 {
        # "Template Separator\n(You can make a copy of, or modify, this frame)"
        n537 = flat-sequence {
          tunnel: [w1327] -> w1316
          tunnel: [w1326] -> w1315
          tunnel: [w1325] -> w1313
          frame #0 {
            w1328 = T2 2 items=["CMD_Eval_Mode_Entry_CC1", "CMD_Eval_Mode_Entry_CC2", "CMD_Eval_Mode_Continue", "CMD_Send_DIAG_Info", "CMD_Enable_Debug_Log ", "CMD_Disable_Debug_Log ", "CMD_Send_Log_Data"] ("Dryer Cmd")
            n538 = local read "Period of STATUS (Counts)"() -> (w1325:dbl)
            n539 = local write "Dryer Status 2 Send"(Dryer_Status_Ctrl."Cycle Completed" ("Dryer Status 2 Send")) -> ()
            n540 = local read "Com:Data"() -> (w1326:string)
            n541 = call "Type Conv - Dryer Cmd to String.vi"("Dryer Cmd"=w1328) -> ("Read String"=w1327:string)  [unwired: 10 in]
            "Wait Restart" <- TRUE ("Wait for Restart")
          }
        }
        n542 = local read "Exit"() -> (w1304:bool)
        n543 = case shown="True" w1304 {
          tunnel: [_ "Exit\n"] -> w1303
          frame #0 {
          }
          frame #1 {
          }
        }
        n544 = call "Counter.vi"() -> ("Count"=w1312:dbl)  [unwired: 11 in]
        n545 = xnode "Match Regular Expression"("input string"=w1315, "regular expression"=w1316) -> ("offset past match"=w1317:i32)  [unwired: 4 in, 4 out]
        n546 = Quotient & Remainder(x=w1312, y=w1313) -> (x-y*floor(x/y)=w1311:dbl)  [unwired: 1 out]
        n547 = Greater Or Equal To 0?(x=w1317) -> (x >= 0?=w1314:bool)
        n548 = Equal To 0?(x=w1311) -> (x = 0?=w1310:bool)
        n549 = Select(t="Send Status\n", s=w1310, f="") -> (s? t:f=w1305:string)
        n550 = case shown="False" w1314 {
          tunnel: ["ReadData\nData: Parse\nWait for Restart" "Timed Dry\nWait for Restart"] -> w1307
          frame #0 {
            n551 = local write "CRC Match"(FALSE ("Wait for Restart")) -> ()
          }
          frame #1 {
            n552 = call "E-Time.vi"() -> ("Elapsed Time (sec)"=w1439:dbl)  [unwired: 9 in, 2 out]
            n553 = local write "Tstart"(w1439) -> ()
            n554 = local write "Wait Restart"(FALSE ("Wait for Restart")) -> ()
            n555 = local write "Com:Data"("" ("Com:Data")) -> ()
          }
        }
        n556 = Wait Until Next ms Multiple(millisecond multiple=u32 1000) -> ()  [unwired: 1 out]
        n557 = Concatenate Strings(w1303, w1305, w1307) -> (w1306:string)
        n558 = call <vilib>:"Add State(s) to Queue__jki_lib_state_machine.vi"("State(s) in Front (\"\")"=w1306, "State(s) in (\"\")"=w1322) -> ("States Out"=w1321:string)  [unwired: 13 in]
      }
    }
    n559 = case shown="True" "Debug" {
      tunnel: w40 -> [w54 w57]
      tunnel: w39 -> [_ w56]
      tunnel: [w54 w55] -> w38
      frame #0 {
      }
      frame #1 {
        n560 = Build Array (concatenate)(w57, w56) -> (w55:string[])
        "State Array" <- w55
      }
    }
    n561 = flat-sequence {
      tunnel: [w59] -> w44
      tunnel: w45 -> [_]
      tunnel: [w58] -> w43
      frame #0 {
        n562 = local read "tStart"() -> (w58:u32)
        n563 = Tick Count (ms)() -> (millisecond timer value=w59:u32)
      }
    }
    n564 = local write "Error Out"(w45) -> ()
    n565 = To Long Integer(number=w44) -> (32bit integer=w42:i32)
    n566 = To Long Integer(number=w43) -> (32bit integer=w41:i32)
  }
  n567 = local read "Debug"() -> (w2:bool)
  n568 = case shown="True" w2 {
    tunnel: w13 -> [_ w1446]
    tunnel: w12 -> [_ w1445]
    frame #0 {
    }
    frame #1 {
      n569 = Subtract(x=w1446, y=w1445) -> (x-y=w1447:i32[])
      "Time Array" <- w1447
      n570 = Delete From Array(array=w1447, length=1, index=0) -> (array with subset deleted=w1448:i32[])  [unwired: 1 out]
      n571 = for {
        tunnel: w1448 -> [w1453] mode=indexing
        tunnel: w1447 -> [w1452] mode=indexing
        tunnel: [w1451] -> w1444 mode=indexing
        n572 = Subtract(x=w1453, y=w1452) -> (x-y=w1451:i32)
      }
      "Tdiff" <- w1444
      n573 = Add Array Elements(numeric array=w1444) -> (sum=→"Total mS":i32)
    }
  }
  n574 = Unbundle By Name(w7) -> ("CRC"=w8:bool)
  n575 = Unbundle By Name(w7) -> ("Error Out Flag"=w6:bool)
  n576 = Bundle By Name(cluster=w14, "status"=w6) -> (w9:errorcluster)
  n577 = disable-structure shown="Enabled" {
    disable-tunnel: [w1468 w1472] -> w10
    disable-tunnel: w9 -> [w1467 w1472]
    disable-tunnel: w8 -> [w1466 _]
    frame #0 {
      # "Patch for double read of ICP"
      n578 = call "Error Bool Enumerator.vi"("Error Enum"=HEWH_Error_Enumeration."GEA2 Send ACK Mismatch", "Error?"=TRUE) -> ("Error Out"=w1455:errorcluster)  [unwired: 7 in]
      n579 = call "Error Bool Enumerator.vi"("Error Enum"=HEWH_Error_Enumeration."GEA2 ETX", "Error?"=TRUE) -> ("Error Out"=w1457:errorcluster)  [unwired: 7 in]
      n580 = Unbundle By Name(w1455) -> ("code"=w1454:i32)
      n581 = Unbundle By Name(w1457) -> ("code"=w1456:i32)
      n582 = Unbundle By Name(w1467) -> ("code"=w1463:i32)
      n583 = Equal?(x=w1463, y=w1456) -> (x = y?=w1464:bool)
      n584 = Equal?(x=w1463, y=w1454) -> (x = y?=w1462:bool)
      n585 = Or(x=w1464, y=w1462) -> (x .or. y?=w1465:bool)
      n586 = And(x=w1466, y=w1465) -> (x .and. y?=w1469:bool)
      n587 = case shown="False" w1469 {
        tunnel: [w1470 errorcluster {"status"=FALSE, "code"=0, "source"="ETX or ACK"} ("Error Out")] -> w1468
        tunnel: w1467 -> [w1470 _]
        frame #0 {
        }
        frame #1 {
        }
      }
    }
    frame #1 {
    }
  }
  "Error Out" <- w10
